vi "MWT.vi"() -> ()   [LabVIEW 2010]
uses:
  MWT_1.3.0_r1035/MultiWorm Tracker v1.3.0/data/MWT.dll
  <vilib>/vision/driver/NI_Vision_Acquisition_Software.lvlib
  <vilib>/vision/Image Controls.llb/IMAQ Image.ctl
  <vilib>/userDefined/High Color/IMAQdx.ctl
panel:
  in  "Turn on external triggering of camera":bool
  in  "User interface display slector":u16(ring)=2 items=["Raw Image", "Memory Image", "Fixed Image", "Nothing"]
  out "Auto-end in (s)":dbl
  out "error out 2":errorcluster
  in  "Minimum time between events(ms)":u32=2000
  in  "custom 1 timing array":dbl[](array[numeric])=[0.0]
  in  "puff timing array":dbl[](array[numeric])=[0.0]
  in  "tap timing array":dbl[](array[numeric])=[0.0]
  in  "custom 2 timing array":dbl[](array[numeric])=[0.0]
  in  "Tap Train Number":i32[][](array[numeric])=[[0, 1]]
  in  "Turn on Background division algorithm":bool
  in  "custom 2 fraction of time between is active":sgl[][](array[numeric])=[[0.0, 0.5]]
  in  "time between custom 2 onset":i32[][](array[numeric])=[[0, 50]]
  in  "custom 1 fraction of time between is active":sgl[][](array[numeric])=[[0.0, 0.5]]
  in  "time between custom 1 onset":i32[][](array[numeric])=[[0, 50]]
  in  "time between puff onset":i32[][](array[numeric])=[[0, 50]]
  in  "puff fraction of time between is active":sgl[][](array[numeric])=[[0.0, 0.5]]
  in  "time between tap onset":i32[][](array[numeric])=[[0, 10]]
  in  "tap fraction of time between is active":sgl[][](array[numeric])=[[0.0, 0.6]]
  in  "Turn on output aggregation?":bool=TRUE
  out "# Custom 2's Delivered":i32
  out "Time until Next Custom 2":dbl caption="No Custom 2s"
  in  "Custom 2 Signal-high lead up":i32=20
  in  "Custom 2 Signal-high duration":i32=50
  in  "Advanced Custom 2 Settings":bool
  in  "Custom 2 Stimulus Method":u16(ring) items=["Fixed Interval"=0, "Exponential Interval"=2, "Custom"=5]
  in  "Custom 2 Number":i32 caption="# of Puff events"
  in  "Custom 2 Interval":dbl caption="Custom Interval (s)"
  in  "Custom 2 Delay":dbl caption="Puff Onset Delay (s)" format="%#_4g"
  in  "Custom 2":bool
  out "Image Data Input Source":T1(ring)
  in  "Number of Image Adaptation Bands":i32=10
  out "error out":errorcluster
  in  "AVI path":path
  out "Auto-start in (s)":dbl
  in  "Auto-start delay (s)":i32
  in  "Raw Image Save Interval (s)":dbl
  in  "IMAQdx camera interface name":T2="cam0"
  out "Query for Interface?":bool=TRUE
  out "last acquired buffer":i32
  in  "Advanced Settings":bool
  out "# Custom 1's Delivered":i32
  out "Time until Next Custom 1":dbl caption="No Custom 1s"
  in  "Custom 1 Signal-high lead up":i32=20
  in  "Custom 1 Signal-high duration":i32=50
  out "Tracker Handle":i32=1
  out "IMAQ Session":refnum<k11>
  in  "Advanced Custom 1 Settings":bool
  in  "Custom 1 Stimulus Method":u16(ring) items=["Fixed Interval"=0, "Exponential Interval"=2, "Custom"=5]
  in  "Custom 1 Number":i32 caption="# of Puff events"
  in  "Custom 1 Interval":dbl caption="Custom Interval (s)"
  in  "Custom 1 Delay":dbl caption="Puff Onset Delay (s)" format="%#_4g"
  in  "Custom 1":bool
  in  "Image Binning":u16(ring)=1 items=["1"=1, "2"=2, "3"=3, "4"=4]
  in  "Contour?":bool
  in  "AFG resource name":refnum<k15>="COM1"
  out "Proccessing loop stopped?":bool
  in  "Object Border":i32=20
  out "AFG Settings":dbl[][](array[numeric])=[[0.0, 10.0, 1.0]]
  out "AFG instrument handle":refnum<k15> caption="instrument handle out"
  in  "Puff Signal-high lead up":i32=20
  in  "Puff Signal-high duration":i32=50
  in  "Frames of Adaptation":i32=10
  out "# Taps Delivered":i32
  out "# Puffs Delivered":i32
  in  "Skeletonize?":bool
  out "ROI Array":dbl[][](array[numeric])=[[0.0, 0.0, 2350.0, 1726.0, 0.0, 0.0]]
  out "Time until Next Puff":dbl caption="No Puffs"
  out "Seconds into Experiment":dbl
  out "Objects Found":i32
  in  "Bit Depth from Camera?":bool=TRUE
  in  "Image Bit Depth":u32=8
  in  "Advanced Puff Settings":bool
  in  "Graph Input 4":u16(ring)=9 items=["# objects", "# objects persisting", "Persistence", "Speed", "Angular Speed", "Length", "Relative Length", "Width", "Relative Width", "Aspect", "Relative Aspect", "Head Or Tail Angle", "Pixel Count"]
  in  "Graph Input 3":u16(ring)=3 items=["# objects", "# objects persisting", "Persistence", "Speed", "Angular Speed", "Length", "Relative Length", "Width", "Relative Width", "Aspect", "Relative Aspect", "Head Or Tail Angle", "Pixel Count"]
  in  "Graph Input 2":u16(ring)=1 items=["# objects", "# objects persisting", "Persistence", "Speed", "Angular Speed", "Length", "Relative Length", "Width", "Relative Width", "Aspect", "Relative Aspect", "Head Or Tail Angle", "Pixel Count"]
  in  "Graph Input":u16(ring) items=["# objects", "# objects persisting", "Persistence", "Speed", "Angular Speed", "Length", "Relative Length", "Width", "Relative Width", "Aspect", "Relative Aspect", "Head or Tail Angle", "Pixel Count"]
  out "XY Graph 4":cluster{sgl, sgl}[](graph)
  out "XY Graph 3":cluster{sgl, sgl}[](graph)
  out "XY Graph 2":cluster{sgl, sgl}[](graph)
  out "XY Graph":cluster{sgl, sgl}[](graph)
  out "Time until Next Tap":dbl caption="No Taps"
  in  "Puff Stimulus Method":u16(ring) items=["Fixed Interval"=0, "Exponential Interval"=2, "Custom"=5]
  in  "Tap Pulse Active downtime":i32=120
  in  "Tap Pulse Active duration":i32=120
  in  "Tap Signal-high duration":i32=100
  in  "Tap Signal-high lead up":i32=20
  out "seconds per frame":sgl
  out "error count":i32
  out "First-call":bool=TRUE
  in  "Run":bool
  in  "Adaptation Rate":i32=5 step=1
  out "Directory Exists?":bool
  in  "IMAQ Camera Interface Name":string="img0"
  in  "Display/Don't Display":bool=TRUE
  in  "What to display":u16(ring)=2 items=["Raw Image", "Memory Image", "Fixed Image"]
  out "Image":T3(plugin-control)
  in  "Stop":bool=TRUE
  in  "Set New Reference Object":bool
  in  "Clear Reference Object(s)":bool
  in  "Set Region of Interest":bool
  in  "Clear Region of Interest":bool
  in  "Load":bool
  in  "Save":bool
  in  "Advanced Tap Settings":bool
  in  "Tap Stimulus Method":u16(ring) items=["Fixed Interval"=0, "Exponential Interval"=2, "Custom"=5]
  in  "Puff Number":i32 caption="# of Puff events"
  in  "Puff Interval":dbl caption="Puff Interval (s)"
  in  "Puff Delay":dbl caption="Puff Onset Delay (s)"
  in  "Tap Number":i32 caption="# of Tap events" step=1
  in  "Tap Interval":dbl caption="Tap Interval (s)"
  in  "Tap Delay":dbl caption="Tap Onset Delay (s)"
  in  "Puff":bool
  in  "Tap":bool
  in  "Experiment Duration (s)":dbl
  in  "Prefix":string
  in  "Path":path
  in  "Object Size hysteresis (%)":dbl=10.0 min=0.5 max=99.5
  in  "Minimum Object Size (pixels)":i32=50
  in  "Maximum Object Size (pixels)":i32=6000
  in  "Fill Hysteresis (%)":dbl=50.0 min=0.5 max=99.5
  in  "Object Contrast (%)":dbl=10.0 min=0.5 max=99.5
  in  "Type of object to track":bool
  # "Display"
  # "Do not display"
  # "Region of Interest"
  # "Reference Object"
  # "Multi-Worm Tracker\nv1.3.0 r1035"
  # "Display"
  # "Object Tracker Settings"
  # "Contrast"
  # "Size"
  # "Bright Objects"
  # "Dark Objects"
  # "Data Ouput Settings"
  # "Stimulus Settings"
  # "On"
  # "On"
  # "On"
  # "On"
  # "Off"
  # "Off"
  # "Off"
  # "Off"
  # "Onset delay (s)"
  # "Interval (s)"
  # "Events (#)"
  # "Configuration"
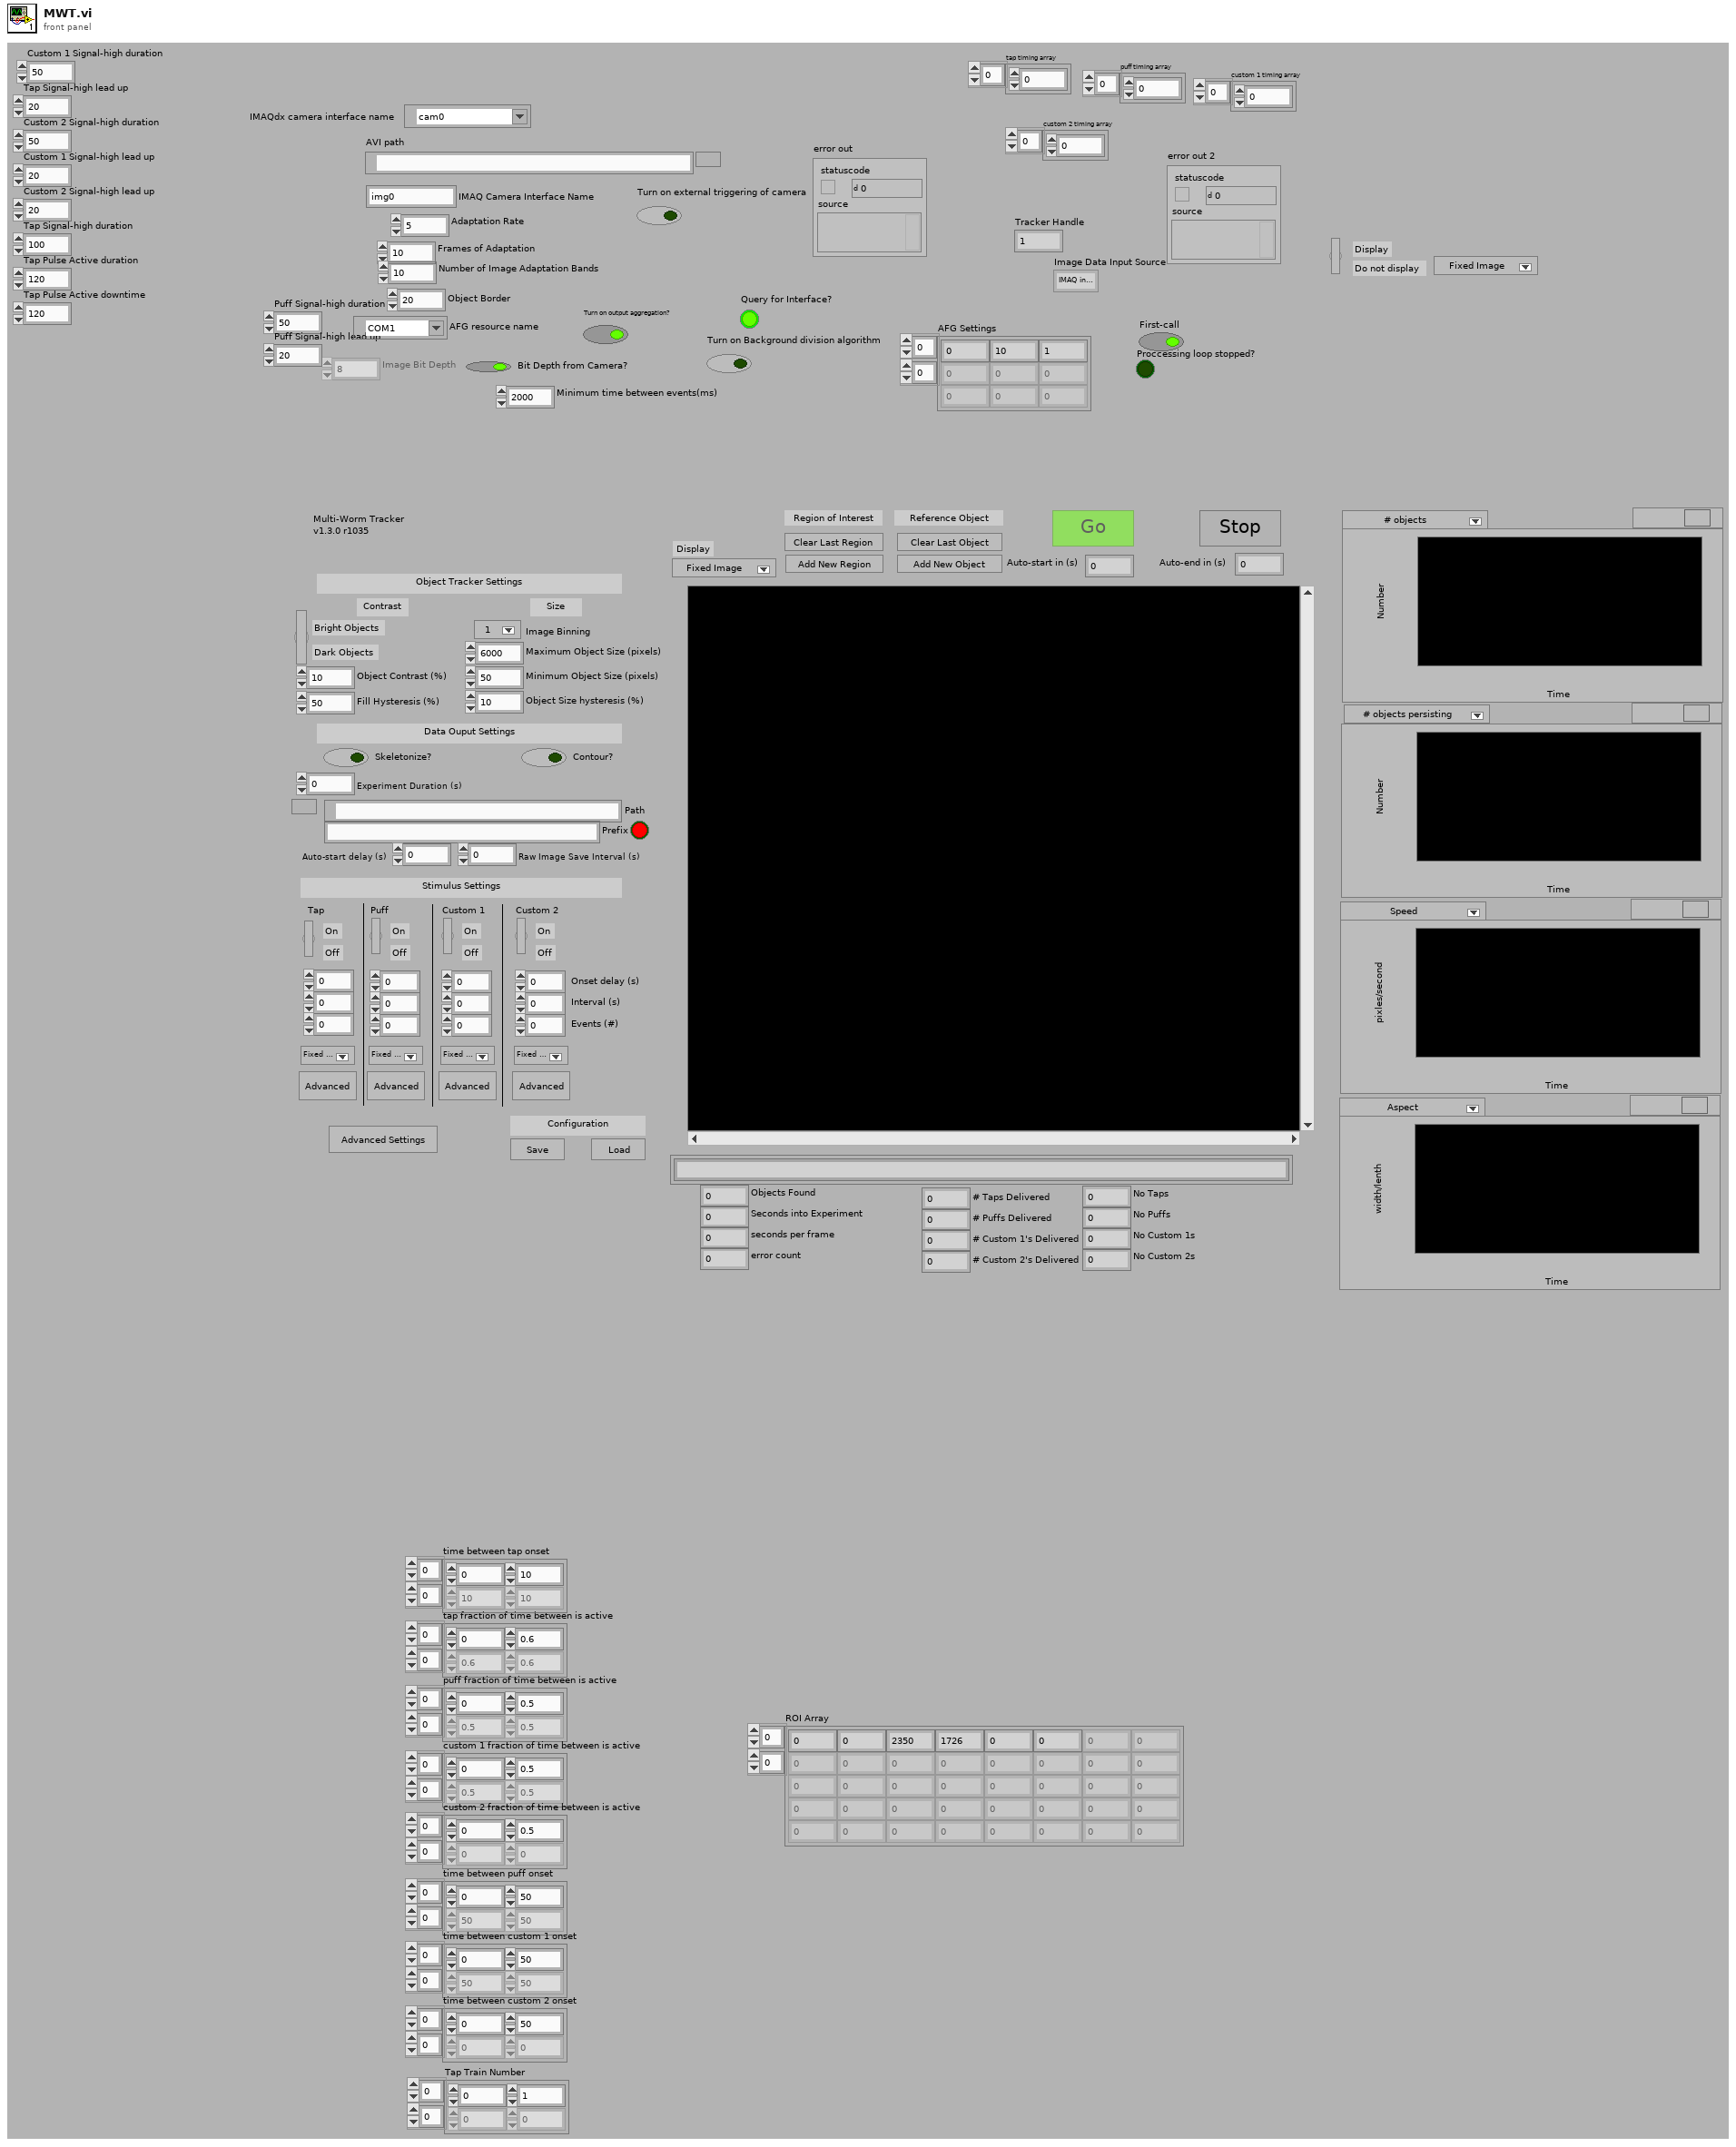
[diagram p1: front panel]
types:
  T1 = enum32{"IMAQ interface", "IMAQdx interface", "AVI file"}
  T2 = typedef "IMAQdx.ctl" = refnum<k21>
  T3 = typedef "IMAQ Image.ctl" = refnum<image>
  T4 = cluster{"Puff":refnum<vi>, "Puff Delay":refnum<vi>, "Puff Interval":refnum<vi>, "Puff Number":refnum<vi>, "Puff Stimulus Method":refnum<vi>}
  T5 = cluster{"Custom 2":refnum<vi>, "Custom 2 Delay":refnum<vi>, "Custom 2 Interval":refnum<vi>, "Custom 2 Number":refnum<vi>, "Custom 2 Stimulus Method":refnum<vi>}
  T6 = cluster{"Custom 1":refnum<vi>, "Custom 1 Delay":refnum<vi>, "Custom 1 Interval":refnum<vi>, "Custom 1 Number":refnum<vi>, "Custom 1 Stimulus Method":refnum<vi>}
  T7 = cluster{"Tap":refnum<vi>, "Tap Delay":refnum<vi>, "Tap Interval":refnum<vi>, "Tap Number":refnum<vi>, "Tap Stimulus Method":refnum<vi>}
  T8 = cluster{cluster{"Tap":refnum<vi>, "Tap Delay":refnum<vi>, "Tap Interval":refnum<vi>, "Tap Number":refnum<vi>, "Tap Stimulus Method":refnum<vi>}, cluster{"Puff":refnum<vi>, "Puff Delay":refnum<vi>, "Puff Interval":refnum<vi>, "Puff Number":refnum<vi>, "Puff Stimulus Method":refnum<vi>}, cluster{"Custom 1":refnum<vi>, "Custom 1 Delay":refnum<vi>, "Custom 1 Interval":refnum<vi>, "Custom 1 Number":refnum<vi>, "Custom 1 Stimulus Method":refnum<vi>}, cluster{"Custom 2":refnum<vi>, "Custom 2 Delay":refnum<vi>, "Custom 2 Interval":refnum<vi>, "Custom 2 Number":refnum<vi>, "Custom 2 Stimulus Method":refnum<vi>}}
  T9 = cluster{"Run":refnum<vi>, "Set Region of Interest":refnum<vi>, "Clear Region of Interest":refnum<vi>, "Clear Reference Object(s)":refnum<vi>, "Set New Reference Object":refnum<vi>, "Advanced Settings":refnum<vi>}
  T10 = cluster{"Path":refnum<vi>, "Prefix":refnum<vi>, "Type of object to track":refnum<vi>, "Object Contrast (%)":refnum<vi>, "Fill Hysteresis (%)":refnum<vi>, "Maximum Object Size (pixels)":refnum<vi>, "Minimum Object Size (pixels)":refnum<vi>, "Object Size hysteresis (%)":refnum<vi>, "Image Binning":refnum<vi>, "Contour?":refnum<vi>, "Skeletonize?":refnum<vi>, "Frames of Adaptation":refnum<vi>, "Adaptation Rate":refnum<vi>, "Object Border":refnum<vi>, "Image Bit Depth":refnum<vi>, "Bit Depth from Camera?":refnum<vi>, "AFG resource name":refnum<vi>, "IMAQ Camera Interface Name":refnum<vi>, "Auto-start delay (s)":refnum<vi>, "Number of Image Adaptation Bands":refnum<vi>, "Experiment Duration (s)":refnum<vi>, "Tap":refnum<vi>, "Tap Delay":refnum<vi>, "Tap Interval":refnum<vi>, "Tap Number":refnum<vi>, "Tap Stimulus Method":refnum<vi>, "Advanced Tap Settings":refnum<vi>, "Puff":refnum<vi>, "Puff Delay":refnum<vi>, "Puff Interval":refnum<vi>, "Puff Number":refnum<vi>, "Puff Stimulus Method":refnum<vi>, "Advanced Puff Settings":refnum<vi>, "Custom 1":refnum<vi>, "Custom 1 Delay":refnum<vi>, "Custom 1 Interval":refnum<vi>, "Custom 1 Number":refnum<vi>, "Custom 1 Stimulus Method":refnum<vi>, "Advanced Custom 1 Settings":refnum<vi>, "puff fraction of time between is active":refnum<vi>, "time between puff onset":refnum<vi>, "tap fraction of time between is active":refnum<vi>, "time between tap onset":refnum<vi>, "Tap Train Number":refnum<vi>, "custom 1 fraction of time between is active":refnum<vi>, "time between custom 1 onset":refnum<vi>, "Custom 2":refnum<vi>, "Custom 2 Delay":refnum<vi>, "Custom 2 Interval":refnum<vi>, "Custom 2 Number":refnum<vi>, "Custom 2 Stimulus Method":refnum<vi>, "Advanced Custom 2 Settings":refnum<vi>, "custom 2 fraction of time between is active":refnum<vi>, "time between custom 2 onset":refnum<vi>, "Save":refnum<vi>, "Load":refnum<vi>, "Raw Image Save Interval (s)":refnum<vi>, "Turn on output aggregation?":refnum<vi>, "Turn on Background division algorithm":refnum<vi>, "Turn on external triggering of camera":refnum<vi>}
  T11 = cluster{cluster{cluster{"Tap":refnum<vi>, "Tap Delay":refnum<vi>, "Tap Interval":refnum<vi>, "Tap Number":refnum<vi>, "Tap Stimulus Method":refnum<vi>}, cluster{"Puff":refnum<vi>, "Puff Delay":refnum<vi>, "Puff Interval":refnum<vi>, "Puff Number":refnum<vi>, "Puff Stimulus Method":refnum<vi>}, cluster{"Custom 1":refnum<vi>, "Custom 1 Delay":refnum<vi>, "Custom 1 Interval":refnum<vi>, "Custom 1 Number":refnum<vi>, "Custom 1 Stimulus Method":refnum<vi>}, cluster{"Custom 2":refnum<vi>, "Custom 2 Delay":refnum<vi>, "Custom 2 Interval":refnum<vi>, "Custom 2 Number":refnum<vi>, "Custom 2 Stimulus Method":refnum<vi>}}, cluster{"Path":refnum<vi>, "Prefix":refnum<vi>, "Type of object to track":refnum<vi>, "Object Contrast (%)":refnum<vi>, "Fill Hysteresis (%)":refnum<vi>, "Maximum Object Size (pixels)":refnum<vi>, "Minimum Object Size (pixels)":refnum<vi>, "Object Size hysteresis (%)":refnum<vi>, "Image Binning":refnum<vi>, "Contour?":refnum<vi>, "Skeletonize?":refnum<vi>, "Frames of Adaptation":refnum<vi>, "Adaptation Rate":refnum<vi>, "Object Border":refnum<vi>, "Image Bit Depth":refnum<vi>, "Bit Depth from Camera?":refnum<vi>, "AFG resource name":refnum<vi>, "IMAQ Camera Interface Name":refnum<vi>, "Auto-start delay (s)":refnum<vi>, "Number of Image Adaptation Bands":refnum<vi>, "Experiment Duration (s)":refnum<vi>, "Tap":refnum<vi>, "Tap Delay":refnum<vi>, "Tap Interval":refnum<vi>, "Tap Number":refnum<vi>, "Tap Stimulus Method":refnum<vi>, "Advanced Tap Settings":refnum<vi>, "Puff":refnum<vi>, "Puff Delay":refnum<vi>, "Puff Interval":refnum<vi>, "Puff Number":refnum<vi>, "Puff Stimulus Method":refnum<vi>, "Advanced Puff Settings":refnum<vi>, "Custom 1":refnum<vi>, "Custom 1 Delay":refnum<vi>, "Custom 1 Interval":refnum<vi>, "Custom 1 Number":refnum<vi>, "Custom 1 Stimulus Method":refnum<vi>, "Advanced Custom 1 Settings":refnum<vi>, "puff fraction of time between is active":refnum<vi>, "time between puff onset":refnum<vi>, "tap fraction of time between is active":refnum<vi>, "time between tap onset":refnum<vi>, "Tap Train Number":refnum<vi>, "custom 1 fraction of time between is active":refnum<vi>, "time between custom 1 onset":refnum<vi>, "Custom 2":refnum<vi>, "Custom 2 Delay":refnum<vi>, "Custom 2 Interval":refnum<vi>, "Custom 2 Number":refnum<vi>, "Custom 2 Stimulus Method":refnum<vi>, "Advanced Custom 2 Settings":refnum<vi>, "custom 2 fraction of time between is active":refnum<vi>, "time between custom 2 onset":refnum<vi>, "Save":refnum<vi>, "Load":refnum<vi>, "Raw Image Save Interval (s)":refnum<vi>, "Turn on output aggregation?":refnum<vi>, "Turn on Background division algorithm":refnum<vi>, "Turn on external triggering of camera":refnum<vi>}, cluster{"Run":refnum<vi>, "Set Region of Interest":refnum<vi>, "Clear Region of Interest":refnum<vi>, "Clear Reference Object(s)":refnum<vi>, "Set New Reference Object":refnum<vi>, "Advanced Settings":refnum<vi>}}
  T12 = cluster{"Value":bool, "Value":dbl, "Value":dbl, "Value":i32, "Value":u16}
  T13 = typedef "AviRefnum.ctl" = refnum<k1>
  T14 = cluster{"IMAQ Session Out":refnum<k11>, "Avi Refnum":T13, "Value":enum32{"IMAQ interface", "IMAQdx interface", "AVI file"}, "Session Out":T2, "Value":bool}
  T15 = cluster{"IMAQ Session":refnum<k11>, "AVI Refnum":refnum<k1>, "Image Data Input Source":enum32{"IMAQ interface", "IMAQdx interface", "AVI file", "MMF File"}, cluster{"IMAQ Name":string, "IMAQDx Session":T2, "AVI/MMF Path":path}, "error?":bool, "use extrenal trigger":bool, "SR handle":u32}
  T16 = enum32{"IMAQ interface", "IMAQdx interface", "AVI file", "MMF File"}
  T17 = cluster{"IMAQ Name":string, "IMAQDx Session":T2, "AVI/MMF Path":path}
  T18 = cluster{"IMAQ Session":refnum<k11>, "AVI Refnum":refnum<k1>, "Image Data Input Source":enum32{"IMAQ interface", "IMAQdx interface", "AVI file", "MMF File"}, "SR handle":u32}
  T19 = cluster{"IMAQ Session":refnum<k11>, "AVI Refnum":refnum<k1>, "Image Data Input Source":enum32{"IMAQ interface", "IMAQdx interface", "AVI file", "MMF File"}, "IMAQDx Session":T2, "Value":bool, "SR handle":u32}
  T20 = typedef "Image Type" = u32
  T21 = cluster{"Value":path, "Value":string, "Value":bool, "Value":dbl, "Value":dbl, "Value":i32, "Value":i32, "Value":dbl, "Value":u16, "Value":bool, "Value":bool, "Value":i32, "Value":i32, "Value":i32, "Value":u32, "Value":i32, "Value":bool}
  T22 = cluster{"AFG Settings":dbl[][], "tap timing array":dbl[], "puff timing array":dbl[], "custom timing array":dbl[], "custom 2 timing array":dbl[], cluster{cluster{"Tap":refnum<vi>, "Tap Delay":refnum<vi>, "Tap Interval":refnum<vi>, "Tap Number":refnum<vi>, "Tap Stimulus Method":refnum<vi>}, cluster{"Puff":refnum<vi>, "Puff Delay":refnum<vi>, "Puff Interval":refnum<vi>, "Puff Number":refnum<vi>, "Puff Stimulus Method":refnum<vi>}, cluster{"Custom 1":refnum<vi>, "Custom 1 Delay":refnum<vi>, "Custom 1 Interval":refnum<vi>, "Custom 1 Number":refnum<vi>, "Custom 1 Stimulus Method":refnum<vi>}, cluster{"Custom 2":refnum<vi>, "Custom 2 Delay":refnum<vi>, "Custom 2 Interval":refnum<vi>, "Custom 2 Number":refnum<vi>, "Custom 2 Stimulus Method":refnum<vi>}}, cluster{"Path":refnum<vi>, "Prefix":refnum<vi>, "Type of object to track":refnum<vi>, "Object Contrast (%)":refnum<vi>, "Fill Hysteresis (%)":refnum<vi>, "Maximum Object Size (pixels)":refnum<vi>, "Minimum Object Size (pixels)":refnum<vi>, "Object Size hysteresis (%)":refnum<vi>, "Image Binning":refnum<vi>, "Contour?":refnum<vi>, "Skeletonize?":refnum<vi>, "Frames of Adaptation":refnum<vi>, "Adaptation Rate":refnum<vi>, "Object Border":refnum<vi>, "Image Bit Depth":refnum<vi>, "Bit Depth from Camera?":refnum<vi>, "AFG resource name":refnum<vi>, "IMAQ Camera Interface Name":refnum<vi>, "Auto-start delay (s)":refnum<vi>, "Number of Image Adaptation Bands":refnum<vi>, "Experiment Duration (s)":refnum<vi>, "Tap":refnum<vi>, "Tap Delay":refnum<vi>, "Tap Interval":refnum<vi>, "Tap Number":refnum<vi>, "Tap Stimulus Method":refnum<vi>, "Advanced Tap Settings":refnum<vi>, "Puff":refnum<vi>, "Puff Delay":refnum<vi>, "Puff Interval":refnum<vi>, "Puff Number":refnum<vi>, "Puff Stimulus Method":refnum<vi>, "Advanced Puff Settings":refnum<vi>, "Custom 1":refnum<vi>, "Custom 1 Delay":refnum<vi>, "Custom 1 Interval":refnum<vi>, "Custom 1 Number":refnum<vi>, "Custom 1 Stimulus Method":refnum<vi>, "Advanced Custom 1 Settings":refnum<vi>, "puff fraction of time between is active":refnum<vi>, "time between puff onset":refnum<vi>, "tap fraction of time between is active":refnum<vi>, "time between tap onset":refnum<vi>, "Tap Train Number":refnum<vi>, "custom 1 fraction of time between is active":refnum<vi>, "time between custom 1 onset":refnum<vi>, "Custom 2":refnum<vi>, "Custom 2 Delay":refnum<vi>, "Custom 2 Interval":refnum<vi>, "Custom 2 Number":refnum<vi>, "Custom 2 Stimulus Method":refnum<vi>, "Advanced Custom 2 Settings":refnum<vi>, "custom 2 fraction of time between is active":refnum<vi>, "time between custom 2 onset":refnum<vi>, "Save":refnum<vi>, "Load":refnum<vi>, "Raw Image Save Interval (s)":refnum<vi>, "Turn on output aggregation?":refnum<vi>, "Turn on Background division algorithm":refnum<vi>, "Turn on external triggering of camera":refnum<vi>}, "output values cluster":cluster{"Value":bool, "Value":dbl, "Value":dbl, "Value":dbl, "Value":u16}, "output values cluster":cluster{"Value":bool, "Value":dbl, "Value":dbl, "Value":dbl, "Value":u16}, "output values cluster":cluster{"Value":bool, "Value":dbl, "Value":dbl, "Value":dbl, "Value":u16}, "output values cluster":cluster{"Value":bool, "Value":dbl, "Value":dbl, "Value":dbl, "Value":u16}}
  T23 = cluster{cluster{"IMAQ Session":refnum<k11>, "AVI Refnum":refnum<k1>, "Image Data Input Source":enum32{"IMAQ interface", "IMAQdx interface", "AVI file", "MMF File"}, "IMAQDx Session":T2, "Value":bool, "SR handle":u32}, "Value":i32, "Value":i32}
  T24 = cluster{"output values cluster":cluster{"Value":bool, "Value":dbl, "Value":dbl, "Value":dbl, "Value":u16}, "Output Array":dbl[], "output values cluster":cluster{"Value":bool, "Value":dbl, "Value":dbl, "Value":dbl, "Value":u16}, "Output Array":dbl[], "output values cluster":cluster{"Value":bool, "Value":dbl, "Value":dbl, "Value":dbl, "Value":u16}, "Output Array":dbl[], "AFG Settings":dbl[][], "output values cluster":cluster{"Value":bool, "Value":dbl, "Value":dbl, "Value":dbl, "Value":u16}, "Output Array":dbl[]}
  T25 = cluster{cluster{cluster{"IMAQ Session":refnum<k11>, "AVI Refnum":refnum<k1>, "Image Data Input Source":enum32{"IMAQ interface", "IMAQdx interface", "AVI file", "MMF File"}, "IMAQDx Session":T2, "Value":bool, "SR handle":u32}, "Value":i32, "Value":i32}, cluster{"Run":refnum<vi>, "Set Region of Interest":refnum<vi>, "Clear Region of Interest":refnum<vi>, "Clear Reference Object(s)":refnum<vi>, "Set New Reference Object":refnum<vi>, "Advanced Settings":refnum<vi>}, "Image Bit Depth":u32}
  T26 = cluster{"Value":bool, "Value":dbl, "Value":dbl, "Value":dbl, "Value":u16}
  T27 = cluster{cluster{cluster{"IMAQ Session":refnum<k11>, "AVI Refnum":refnum<k1>, "Image Data Input Source":enum32{"IMAQ interface", "IMAQdx interface", "AVI file", "MMF File"}, "IMAQDx Session":T2, "Value":bool, "SR handle":u32}, "Value":i32, "Value":i32}, cluster{"Path":refnum<vi>, "Prefix":refnum<vi>, "Type of object to track":refnum<vi>, "Object Contrast (%)":refnum<vi>, "Fill Hysteresis (%)":refnum<vi>, "Maximum Object Size (pixels)":refnum<vi>, "Minimum Object Size (pixels)":refnum<vi>, "Object Size hysteresis (%)":refnum<vi>, "Image Binning":refnum<vi>, "Contour?":refnum<vi>, "Skeletonize?":refnum<vi>, "Frames of Adaptation":refnum<vi>, "Adaptation Rate":refnum<vi>, "Object Border":refnum<vi>, "Image Bit Depth":refnum<vi>, "Bit Depth from Camera?":refnum<vi>, "AFG resource name":refnum<vi>, "IMAQ Camera Interface Name":refnum<vi>, "Auto-start delay (s)":refnum<vi>, "Number of Image Adaptation Bands":refnum<vi>, "Experiment Duration (s)":refnum<vi>, "Tap":refnum<vi>, "Tap Delay":refnum<vi>, "Tap Interval":refnum<vi>, "Tap Number":refnum<vi>, "Tap Stimulus Method":refnum<vi>, "Advanced Tap Settings":refnum<vi>, "Puff":refnum<vi>, "Puff Delay":refnum<vi>, "Puff Interval":refnum<vi>, "Puff Number":refnum<vi>, "Puff Stimulus Method":refnum<vi>, "Advanced Puff Settings":refnum<vi>, "Custom 1":refnum<vi>, "Custom 1 Delay":refnum<vi>, "Custom 1 Interval":refnum<vi>, "Custom 1 Number":refnum<vi>, "Custom 1 Stimulus Method":refnum<vi>, "Advanced Custom 1 Settings":refnum<vi>, "puff fraction of time between is active":refnum<vi>, "time between puff onset":refnum<vi>, "tap fraction of time between is active":refnum<vi>, "time between tap onset":refnum<vi>, "Tap Train Number":refnum<vi>, "custom 1 fraction of time between is active":refnum<vi>, "time between custom 1 onset":refnum<vi>, "Custom 2":refnum<vi>, "Custom 2 Delay":refnum<vi>, "Custom 2 Interval":refnum<vi>, "Custom 2 Number":refnum<vi>, "Custom 2 Stimulus Method":refnum<vi>, "Advanced Custom 2 Settings":refnum<vi>, "custom 2 fraction of time between is active":refnum<vi>, "time between custom 2 onset":refnum<vi>, "Save":refnum<vi>, "Load":refnum<vi>, "Raw Image Save Interval (s)":refnum<vi>, "Turn on output aggregation?":refnum<vi>, "Turn on Background division algorithm":refnum<vi>, "Turn on external triggering of camera":refnum<vi>}, "ROI Array":dbl[][], "settings value cluster":cluster{"Value":path, "Value":string, "Value":bool, "Value":dbl, "Value":dbl, "Value":i32, "Value":i32, "Value":dbl, "Value":u16, "Value":bool, "Value":bool, "Value":i32, "Value":i32, "Value":i32, "Value":u32, "Value":i32, "Value":bool}, "AFG Settings":dbl[][], "Output Array":dbl[], "Output Array":dbl[], "Output Array":dbl[], "Output Array":dbl[]}
  T28 = cluster{"Output  ROI Array":dbl[][], "settings value cluster":cluster{"Value":path, "Value":string, "Value":bool, "Value":dbl, "Value":dbl, "Value":i32, "Value":i32, "Value":dbl, "Value":u16, "Value":bool, "Value":bool, "Value":i32, "Value":i32, "Value":i32, "Value":u32, "Value":i32, "Value":bool}, "AFG Settings":dbl[][], "tap timing array":dbl[], "puff timing array":dbl[], "custom timing array":dbl[], "custom 2 timing array":dbl[]}
  T29 = cluster{cluster{"Path":refnum<vi>, "Prefix":refnum<vi>, "Type of object to track":refnum<vi>, "Object Contrast (%)":refnum<vi>, "Fill Hysteresis (%)":refnum<vi>, "Maximum Object Size (pixels)":refnum<vi>, "Minimum Object Size (pixels)":refnum<vi>, "Object Size hysteresis (%)":refnum<vi>, "Image Binning":refnum<vi>, "Contour?":refnum<vi>, "Skeletonize?":refnum<vi>, "Frames of Adaptation":refnum<vi>, "Adaptation Rate":refnum<vi>, "Object Border":refnum<vi>, "Image Bit Depth":refnum<vi>, "Bit Depth from Camera?":refnum<vi>, "AFG resource name":refnum<vi>, "IMAQ Camera Interface Name":refnum<vi>, "Auto-start delay (s)":refnum<vi>, "Number of Image Adaptation Bands":refnum<vi>, "Experiment Duration (s)":refnum<vi>, "Tap":refnum<vi>, "Tap Delay":refnum<vi>, "Tap Interval":refnum<vi>, "Tap Number":refnum<vi>, "Tap Stimulus Method":refnum<vi>, "Advanced Tap Settings":refnum<vi>, "Puff":refnum<vi>, "Puff Delay":refnum<vi>, "Puff Interval":refnum<vi>, "Puff Number":refnum<vi>, "Puff Stimulus Method":refnum<vi>, "Advanced Puff Settings":refnum<vi>, "Custom 1":refnum<vi>, "Custom 1 Delay":refnum<vi>, "Custom 1 Interval":refnum<vi>, "Custom 1 Number":refnum<vi>, "Custom 1 Stimulus Method":refnum<vi>, "Advanced Custom 1 Settings":refnum<vi>, "puff fraction of time between is active":refnum<vi>, "time between puff onset":refnum<vi>, "tap fraction of time between is active":refnum<vi>, "time between tap onset":refnum<vi>, "Tap Train Number":refnum<vi>, "custom 1 fraction of time between is active":refnum<vi>, "time between custom 1 onset":refnum<vi>, "Custom 2":refnum<vi>, "Custom 2 Delay":refnum<vi>, "Custom 2 Interval":refnum<vi>, "Custom 2 Number":refnum<vi>, "Custom 2 Stimulus Method":refnum<vi>, "Advanced Custom 2 Settings":refnum<vi>, "custom 2 fraction of time between is active":refnum<vi>, "time between custom 2 onset":refnum<vi>, "Save":refnum<vi>, "Load":refnum<vi>, "Raw Image Save Interval (s)":refnum<vi>, "Turn on output aggregation?":refnum<vi>, "Turn on Background division algorithm":refnum<vi>, "Turn on external triggering of camera":refnum<vi>}, cluster{"IMAQ Session":refnum<k11>, "AVI Refnum":refnum<k1>, "Image Data Input Source":enum32{"IMAQ interface", "IMAQdx interface", "AVI file", "MMF File"}, "IMAQDx Session":T2, "Value":bool, "SR handle":u32}}
  T30 = cluster{cluster{cluster{"IMAQ Session":refnum<k11>, "AVI Refnum":refnum<k1>, "Image Data Input Source":enum32{"IMAQ interface", "IMAQdx interface", "AVI file", "MMF File"}, "IMAQDx Session":T2, "Value":bool, "SR handle":u32}, "Value":i32, "Value":i32}, "Image Binning":u16, "Value":u16}
  T31 = cluster{"Acquired Buffer Number":i32, "return type":i32, "destination":i16[][]}
  T32 = cluster{cluster{cluster{"IMAQ Session":refnum<k11>, "AVI Refnum":refnum<k1>, "Image Data Input Source":enum32{"IMAQ interface", "IMAQdx interface", "AVI file", "MMF File"}, "IMAQDx Session":T2, "Value":bool, "SR handle":u32}, "Value":i32, "Value":i32}, "ROI Array":dbl[][], "Value":bool, cluster{"Path":refnum<vi>, "Prefix":refnum<vi>, "Type of object to track":refnum<vi>, "Object Contrast (%)":refnum<vi>, "Fill Hysteresis (%)":refnum<vi>, "Maximum Object Size (pixels)":refnum<vi>, "Minimum Object Size (pixels)":refnum<vi>, "Object Size hysteresis (%)":refnum<vi>, "Image Binning":refnum<vi>, "Contour?":refnum<vi>, "Skeletonize?":refnum<vi>, "Frames of Adaptation":refnum<vi>, "Adaptation Rate":refnum<vi>, "Object Border":refnum<vi>, "Image Bit Depth":refnum<vi>, "Bit Depth from Camera?":refnum<vi>, "AFG resource name":refnum<vi>, "IMAQ Camera Interface Name":refnum<vi>, "Auto-start delay (s)":refnum<vi>, "Number of Image Adaptation Bands":refnum<vi>, "Experiment Duration (s)":refnum<vi>, "Tap":refnum<vi>, "Tap Delay":refnum<vi>, "Tap Interval":refnum<vi>, "Tap Number":refnum<vi>, "Tap Stimulus Method":refnum<vi>, "Advanced Tap Settings":refnum<vi>, "Puff":refnum<vi>, "Puff Delay":refnum<vi>, "Puff Interval":refnum<vi>, "Puff Number":refnum<vi>, "Puff Stimulus Method":refnum<vi>, "Advanced Puff Settings":refnum<vi>, "Custom 1":refnum<vi>, "Custom 1 Delay":refnum<vi>, "Custom 1 Interval":refnum<vi>, "Custom 1 Number":refnum<vi>, "Custom 1 Stimulus Method":refnum<vi>, "Advanced Custom 1 Settings":refnum<vi>, "puff fraction of time between is active":refnum<vi>, "time between puff onset":refnum<vi>, "tap fraction of time between is active":refnum<vi>, "time between tap onset":refnum<vi>, "Tap Train Number":refnum<vi>, "custom 1 fraction of time between is active":refnum<vi>, "time between custom 1 onset":refnum<vi>, "Custom 2":refnum<vi>, "Custom 2 Delay":refnum<vi>, "Custom 2 Interval":refnum<vi>, "Custom 2 Number":refnum<vi>, "Custom 2 Stimulus Method":refnum<vi>, "Advanced Custom 2 Settings":refnum<vi>, "custom 2 fraction of time between is active":refnum<vi>, "time between custom 2 onset":refnum<vi>, "Save":refnum<vi>, "Load":refnum<vi>, "Raw Image Save Interval (s)":refnum<vi>, "Turn on output aggregation?":refnum<vi>, "Turn on Background division algorithm":refnum<vi>, "Turn on external triggering of camera":refnum<vi>}, cluster{"Run":refnum<vi>, "Set Region of Interest":refnum<vi>, "Clear Region of Interest":refnum<vi>, "Clear Reference Object(s)":refnum<vi>, "Set New Reference Object":refnum<vi>, "Advanced Settings":refnum<vi>}, "Directory Exists?":refnum<vi>}
  T33 = cluster{cluster{"IMAQ Session":refnum<k11>, "AVI Refnum":refnum<k1>, "Image Data Input Source":enum32{"IMAQ interface", "IMAQdx interface", "AVI file", "MMF File"}, "IMAQDx Session":T2, "Value":bool, "SR handle":u32}, i32}
  T34 = cluster{"tap timing array":dbl[], "puff timing array":dbl[], "custom timing array":dbl[], "custom 2 timing array":dbl[]}
  T35 = cluster{"width":u32, "height":u32, "framesPerSecond":u32, "compressionFilter":string, "hasData":bool}
  T36 = cluster{cluster{"IMAQ Session":refnum<k11>, "AVI Refnum":refnum<k1>, "Image Data Input Source":enum32{"IMAQ interface", "IMAQdx interface", "AVI file", "MMF File"}, "IMAQDx Session":T2, "Value":bool, "SR handle":u32}, "Value":i32}
  T37 = cluster{cluster{cluster{"IMAQ Session":refnum<k11>, "AVI Refnum":refnum<k1>, "Image Data Input Source":enum32{"IMAQ interface", "IMAQdx interface", "AVI file", "MMF File"}, "IMAQDx Session":T2, "Value":bool, "SR handle":u32}, "Value":i32}, "Value":i32, "Value":i32, "Value":u16, "Image":T3}
  T38 = cluster{cluster{"IMAQ Session":refnum<k11>, "AVI Refnum":refnum<k1>, "Image Data Input Source":enum32{"IMAQ interface", "IMAQdx interface", "AVI file", "MMF File"}, "IMAQDx Session":T2, "Value":bool, "SR handle":u32}, "Acquired Buffer Number":u32}
  T39 = cluster{cluster{"Path":refnum<vi>, "Prefix":refnum<vi>, "Type of object to track":refnum<vi>, "Object Contrast (%)":refnum<vi>, "Fill Hysteresis (%)":refnum<vi>, "Maximum Object Size (pixels)":refnum<vi>, "Minimum Object Size (pixels)":refnum<vi>, "Object Size hysteresis (%)":refnum<vi>, "Image Binning":refnum<vi>, "Contour?":refnum<vi>, "Skeletonize?":refnum<vi>, "Frames of Adaptation":refnum<vi>, "Adaptation Rate":refnum<vi>, "Object Border":refnum<vi>, "Image Bit Depth":refnum<vi>, "Bit Depth from Camera?":refnum<vi>, "AFG resource name":refnum<vi>, "IMAQ Camera Interface Name":refnum<vi>, "Auto-start delay (s)":refnum<vi>, "Number of Image Adaptation Bands":refnum<vi>, "Experiment Duration (s)":refnum<vi>, "Tap":refnum<vi>, "Tap Delay":refnum<vi>, "Tap Interval":refnum<vi>, "Tap Number":refnum<vi>, "Tap Stimulus Method":refnum<vi>, "Advanced Tap Settings":refnum<vi>, "Puff":refnum<vi>, "Puff Delay":refnum<vi>, "Puff Interval":refnum<vi>, "Puff Number":refnum<vi>, "Puff Stimulus Method":refnum<vi>, "Advanced Puff Settings":refnum<vi>, "Custom 1":refnum<vi>, "Custom 1 Delay":refnum<vi>, "Custom 1 Interval":refnum<vi>, "Custom 1 Number":refnum<vi>, "Custom 1 Stimulus Method":refnum<vi>, "Advanced Custom 1 Settings":refnum<vi>, "puff fraction of time between is active":refnum<vi>, "time between puff onset":refnum<vi>, "tap fraction of time between is active":refnum<vi>, "time between tap onset":refnum<vi>, "Tap Train Number":refnum<vi>, "custom 1 fraction of time between is active":refnum<vi>, "time between custom 1 onset":refnum<vi>, "Custom 2":refnum<vi>, "Custom 2 Delay":refnum<vi>, "Custom 2 Interval":refnum<vi>, "Custom 2 Number":refnum<vi>, "Custom 2 Stimulus Method":refnum<vi>, "Advanced Custom 2 Settings":refnum<vi>, "custom 2 fraction of time between is active":refnum<vi>, "time between custom 2 onset":refnum<vi>, "Save":refnum<vi>, "Load":refnum<vi>, "Raw Image Save Interval (s)":refnum<vi>, "Turn on output aggregation?":refnum<vi>, "Turn on Background division algorithm":refnum<vi>, "Turn on external triggering of camera":refnum<vi>}, "appended path":path, "ROI Array":dbl[][], "AFG Settings":dbl[][], "tap timing array":dbl[], "puff timing array":dbl[], "custom timing array":dbl[], "custom 2 timing array":dbl[]}
  T40 = cluster{cluster{"IMAQ Session":refnum<k11>, "AVI Refnum":refnum<k1>, "Image Data Input Source":enum32{"IMAQ interface", "IMAQdx interface", "AVI file", "MMF File"}, "IMAQDx Session":T2, "Value":bool, "SR handle":u32}, "Acquired Buffer Number":i32}
  T41 = cluster{"Graph Input":refnum<vi>, "Graph Input 2":refnum<vi>, "Graph Input 3":refnum<vi>, "Graph Input 4":refnum<vi>, "XY Graph":refnum<vi>, "XY Graph 2":refnum<vi>, "XY Graph 3":refnum<vi>, "XY Graph 4":refnum<vi>}
  T42 = cluster{"Value":sgl[][], "Value":i32[][], "Value":i32[][]}
  T43 = cluster{cluster{sgl, sgl}[], cluster{sgl, sgl}[], cluster{sgl, sgl}[], cluster{sgl, sgl}[], cluster{sgl, sgl}[], cluster{sgl, sgl}[], cluster{sgl, sgl}[], cluster{sgl, sgl}[], cluster{sgl, sgl}[], cluster{sgl, sgl}[], cluster{sgl, sgl}[], cluster{sgl, sgl}[], cluster{sgl, sgl}[]}
  T44 = cluster{"custom timing array":dbl[], i32, i32, "Value":bool, i32, "stimulus settings":cluster{"outy3":sgl, "outy3":i32}}
  T45 = cluster{"custom 2 timing array":dbl[], i32, i32, "Value":bool, i32, "stimulus settings":cluster{"outy3":sgl, "outy3":i32}}
  T46 = cluster{"puff timing array":dbl[], i32, i32, "Value":bool, i32, "stimulus settings":cluster{"outy3":sgl, "outy3":i32}}
  T47 = cluster{"tap timing array":dbl[], i32, i32, "Value":bool, i32, "stimulus settings":cluster{"outy3":sgl, "outy3":i32, "Value":i32}}
  T48 = cluster{u32, "millisecond timer value":u32, "millisecond timer value":u32, "Value":u32}
  T49 = cluster{cluster{u32, "millisecond timer value":u32, "millisecond timer value":u32, "Value":u32}, "Time until Next Tap":refnum<vi>, cluster{"tap timing array":dbl[], i32, i32, "Value":bool, i32, "stimulus settings":cluster{"outy3":sgl, "outy3":i32, "Value":i32}}}
  T50 = cluster{cluster{u32, "millisecond timer value":u32, "millisecond timer value":u32, "Value":u32}, "Time until Next Puff":refnum<vi>, cluster{"puff timing array":dbl[], i32, i32, "Value":bool, i32, "stimulus settings":cluster{"outy3":sgl, "outy3":i32}}}
  T51 = cluster{cluster{u32, "millisecond timer value":u32, "millisecond timer value":u32, "Value":u32}, "Time until Next Custom 1":refnum<vi>, cluster{"custom timing array":dbl[], i32, i32, "Value":bool, i32, "stimulus settings":cluster{"outy3":sgl, "outy3":i32}}}
  T52 = cluster{cluster{u32, "millisecond timer value":u32, "millisecond timer value":u32, "Value":u32}, "Time until Next Custom 2":refnum<vi>, cluster{"custom 2 timing array":dbl[], i32, i32, "Value":bool, i32, "stimulus settings":cluster{"outy3":sgl, "outy3":i32}}}
  T53 = cluster{"millisecond timer value":u32, "millisecond timer value":u32, i32, sgl, "Data Cluster":cluster{cluster{sgl, sgl}[], cluster{sgl, sgl}[], cluster{sgl, sgl}[], cluster{sgl, sgl}[], cluster{sgl, sgl}[], cluster{sgl, sgl}[], cluster{sgl, sgl}[], cluster{sgl, sgl}[], cluster{sgl, sgl}[], cluster{sgl, sgl}[], cluster{sgl, sgl}[], cluster{sgl, sgl}[], cluster{sgl, sgl}[]}, "Value":i32, cluster{"Graph Input":refnum<vi>, "Graph Input 2":refnum<vi>, "Graph Input 3":refnum<vi>, "Graph Input 4":refnum<vi>, "XY Graph":refnum<vi>, "XY Graph 2":refnum<vi>, "XY Graph 3":refnum<vi>, "XY Graph 4":refnum<vi>}}
  T54 = cluster{i32, "Tap Number":i32, "Elapsed Time":i32}
  T55 = cluster{"Elapsed Time":i32, "Data Cluster":cluster{cluster{sgl, sgl}[], cluster{sgl, sgl}[], cluster{sgl, sgl}[], cluster{sgl, sgl}[], cluster{sgl, sgl}[], cluster{sgl, sgl}[], cluster{sgl, sgl}[], cluster{sgl, sgl}[], cluster{sgl, sgl}[], cluster{sgl, sgl}[], cluster{sgl, sgl}[], cluster{sgl, sgl}[], cluster{sgl, sgl}[]}}
  T56 = cluster{i32, "Value":i32, "Value":u16, sgl, "Value":u16, "Value":bool, "Value":u32, "Image Out":T3, "Image Pixels (I16)":i16[][], i32[]}
  T57 = cluster{"return value":i32, "return value":i32, "Image Pixels (I16) out":i16[][], "coordinates":i32[]}
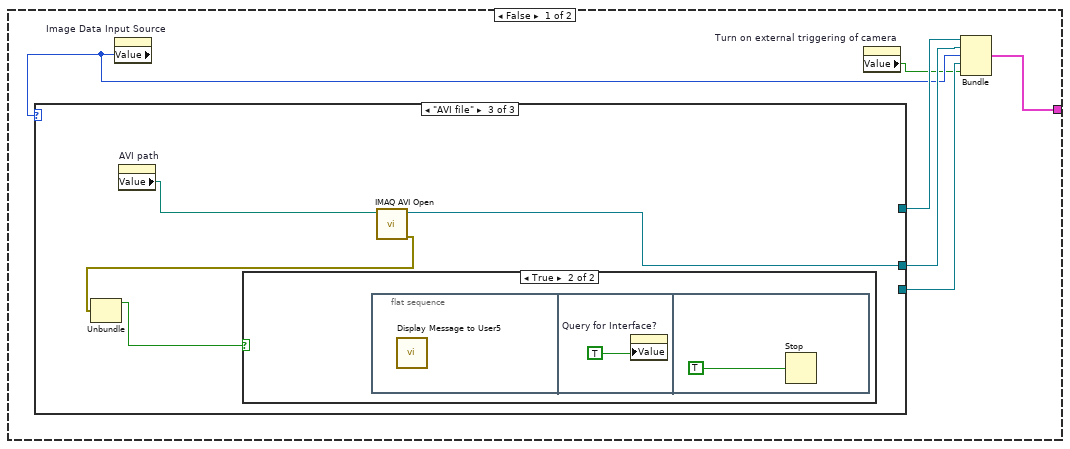
[diagram p2: hidden frame]
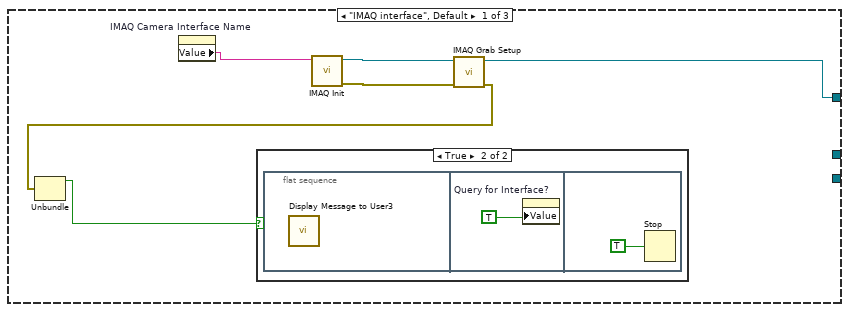
[diagram p3: hidden frame]
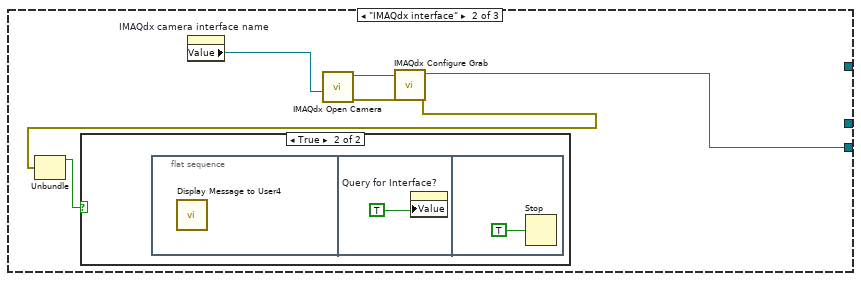
[diagram p5: hidden frame]
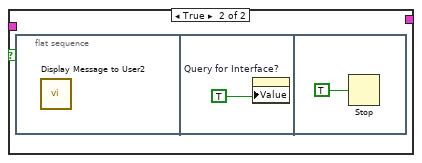
[diagram p8: hidden frame]
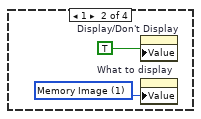
[diagram p11: hidden frame]
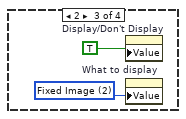
[diagram p12: hidden frame]
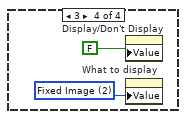
[diagram p13: hidden frame]
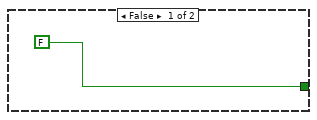
[diagram p14: hidden frame]
diagram:
  w3 = cluster{sgl, sgl}[] [] ("XY Graph")
  w24 = 0
  # "Stimulus counter trigger arrays"
  # "Stimulus event timing arrays"
  # "Copyright (C) 2007 - 2010 Howard Hughes Medical Institute\nCopyright (C) 2007 - 2010 Rex A. Kerr, Nicholas A. Swierczek\n \nThis file is a part of the Multi-Worm Tracker and is distributed under the\nterms of the GNU Lesser General Public Licence version 2.1 (LGPL 2.1).\nFor details, see GPL2.txt and LGPL2.1.txt, or http://www.gnu.org/licences\n \nTo contact the authors, email kerrlab@users.sourceforge.net."
  # "Device Start Timing Control"
  # "Main Controls Cluster"
  # "Assorted buttons for advanced settings/ROI/reference objects"
  # "Stimulus Timing Controls"
  # "Exp. Duration"
  # "Array of ROIs"
  # "Statistics data controls"
  # "Display Controls; \ndisplay type and display on/off toggle"
  # "Settigns-related buttons"
  # "ROI-related buttons"
  # "Reference Object-related buttons"
  # "Overall control buttons"
  # "Image Bit Depth Control"
  # "Function Generator Settings"
  # "Image/Tracking Parameters"
  # "Blob Tracking Parameters"
  # "State variables"
  # "Images"
  # "Hardware System names/handles"
  # "Graph FP objects and controls"
  # "Stimulus delivery control parameters"
  # "Stimulus control signal parameters"
  # "Front panel indicators"
  # "Data output parameters"
  # "References to the front panel controls"
  n1 = control-ref of="AFG resource name"() -> (w70:refnum<vi>)
  n2 = control-ref of="Turn on Background division algorithm"() -> (w4:refnum<vi>)
  n3 = control-ref of="Turn on external triggering of camera"() -> (w2:refnum<vi>)
  n4 = control-ref of="Turn on output aggregation?"() -> (w5:refnum<vi>)
  n5 = control-ref of="Run"() -> (w101:refnum<vi>)
  n6 = control-ref of="Save"() -> (w16:refnum<vi>)
  n7 = control-ref of="Load"() -> (w17:refnum<vi>)
  n8 = control-ref of="Set Region of Interest"() -> (w115:refnum<vi>)
  n9 = control-ref of="Clear Region of Interest"() -> (w118:refnum<vi>)
  n10 = control-ref of="Clear Reference Object(s)"() -> (w117:refnum<vi>)
  n11 = control-ref of="Set New Reference Object"() -> (w116:refnum<vi>)
  n12 = control-ref of="Advanced Settings"() -> (w87:refnum<vi>)
  n13 = control-ref of="Custom 2"() -> (w8:refnum<vi>)
  n14 = control-ref of="Advanced Custom 2 Settings"() -> (w13:refnum<vi>)
  n15 = control-ref of="Tap"() -> (w49:refnum<vi>)
  n16 = control-ref of="Advanced Tap Settings"() -> (w44:refnum<vi>)
  n17 = control-ref of="Puff"() -> (w43:refnum<vi>)
  n18 = control-ref of="Advanced Puff Settings"() -> (w38:refnum<vi>)
  n19 = control-ref of="Custom 1"() -> (w37:refnum<vi>)
  n20 = control-ref of="Advanced Custom 1 Settings"() -> (w32:refnum<vi>)
  n21 = control-ref of="Type of object to track"() -> (w84:refnum<vi>)
  n22 = control-ref of="Contour?"() -> (w77:refnum<vi>)
  n23 = control-ref of="Skeletonize?"() -> (w76:refnum<vi>)
  n24 = control-ref of="Bit Depth from Camera?"() -> (w71:refnum<vi>)
  n25 = control-ref of="Raw Image Save Interval (s)"() -> (w7:refnum<vi>)
  n26 = control-ref of="Custom 2"() -> (w19:refnum<vi>)
  n27 = control-ref of="Custom 2 Delay"() -> (w9:refnum<vi>)
  n28 = control-ref of="Custom 2 Interval"() -> (w10:refnum<vi>)
  n29 = control-ref of="Custom 2 Number"() -> (w11:refnum<vi>)
  n30 = control-ref of="Custom 1"() -> (w92:refnum<vi>)
  n31 = control-ref of="Auto-start delay (s)"() -> (w52:refnum<vi>)
  n32 = control-ref of="Number of Image Adaptation Bands"() -> (w51:refnum<vi>)
  n33 = control-ref of="Experiment Duration (s)"() -> (w50:refnum<vi>)
  n34 = control-ref of="Tap Delay"() -> (w48:refnum<vi>)
  n35 = control-ref of="Tap Interval"() -> (w47:refnum<vi>)
  n36 = control-ref of="Tap Number"() -> (w46:refnum<vi>)
  n37 = control-ref of="Puff Delay"() -> (w42:refnum<vi>)
  n38 = control-ref of="Puff Interval"() -> (w41:refnum<vi>)
  n39 = control-ref of="Puff Number"() -> (w40:refnum<vi>)
  n40 = control-ref of="Custom 1 Delay"() -> (w36:refnum<vi>)
  n41 = control-ref of="Custom 1 Interval"() -> (w35:refnum<vi>)
  n42 = control-ref of="Custom 1 Number"() -> (w34:refnum<vi>)
  n43 = control-ref of="Object Contrast (%)"() -> (w83:refnum<vi>)
  n44 = control-ref of="Fill Hysteresis (%)"() -> (w82:refnum<vi>)
  n45 = control-ref of="Maximum Object Size (pixels)"() -> (w81:refnum<vi>)
  n46 = control-ref of="Minimum Object Size (pixels)"() -> (w80:refnum<vi>)
  n47 = control-ref of="Object Size hysteresis (%)"() -> (w79:refnum<vi>)
  n48 = control-ref of="Frames of Adaptation"() -> (w75:refnum<vi>)
  n49 = control-ref of="Adaptation Rate"() -> (w74:refnum<vi>)
  n50 = control-ref of="Object Border"() -> (w73:refnum<vi>)
  n51 = control-ref of="Image Bit Depth"() -> (w72:refnum<vi>)
  n52 = control-ref of="Puff"() -> (w109:refnum<vi>)
  n53 = control-ref of="custom 2 fraction of time between is active"() -> (w14:refnum<vi>)
  n54 = control-ref of="time between custom 2 onset"() -> (w15:refnum<vi>)
  n55 = control-ref of="Prefix"() -> (w85:refnum<vi>)
  n56 = control-ref of="IMAQ Camera Interface Name"() -> (w69:refnum<vi>)
  n57 = control-ref of="puff fraction of time between is active"() -> (w31:refnum<vi>)
  n58 = control-ref of="time between puff onset"() -> (w30:refnum<vi>)
  n59 = control-ref of="tap fraction of time between is active"() -> (w29:refnum<vi>)
  n60 = control-ref of="time between tap onset"() -> (w28:refnum<vi>)
  n61 = control-ref of="Tap Train Number"() -> (w27:refnum<vi>)
  n62 = control-ref of="custom 1 fraction of time between is active"() -> (w26:refnum<vi>)
  n63 = control-ref of="time between custom 1 onset"() -> (w25:refnum<vi>)
  n64 = control-ref of="Custom 2 Interval"() -> (w21:refnum<vi>)
  n65 = control-ref of="Custom 2 Number"() -> (w22:refnum<vi>)
  n66 = control-ref of="Custom 1 Interval"() -> (w90:refnum<vi>)
  n67 = control-ref of="Custom 1 Number"() -> (w89:refnum<vi>)
  n68 = control-ref of="Custom 2 Delay"() -> (w20:refnum<vi>)
  n69 = control-ref of="Custom 2 Stimulus Method"() -> (w12:refnum<vi>)
  n70 = control-ref of="Tap"() -> (w113:refnum<vi>)
  n71 = control-ref of="Custom 1 Delay"() -> (w91:refnum<vi>)
  n72 = control-ref of="Path"() -> (w86:refnum<vi>)
  n73 = control-ref of="Tap Stimulus Method"() -> (w45:refnum<vi>)
  n74 = control-ref of="Puff Stimulus Method"() -> (w39:refnum<vi>)
  n75 = control-ref of="Custom 1 Stimulus Method"() -> (w33:refnum<vi>)
  n76 = control-ref of="Image Binning"() -> (w78:refnum<vi>)
  n77 = control-ref of="Puff Delay"() -> (w108:refnum<vi>)
  n78 = control-ref of="Puff Interval"() -> (w107:refnum<vi>)
  n79 = control-ref of="Puff Number"() -> (w106:refnum<vi>)
  n80 = control-ref of="Custom 2 Stimulus Method"() -> (w23:refnum<vi>)
  n81 = control-ref of="Tap Delay"() -> (w112:refnum<vi>)
  n82 = control-ref of="Tap Interval"() -> (w111:refnum<vi>)
  n83 = control-ref of="Tap Number"() -> (w110:refnum<vi>)
  n84 = control-ref of="Custom 1 Stimulus Method"() -> (w88:refnum<vi>)
  n85 = control-ref of="Puff Stimulus Method"() -> (w104:refnum<vi>)
  n86 = control-ref of="Tap Stimulus Method"() -> (w105:refnum<vi>)
  n87 = Bundle("Puff"=w109, "Puff Delay"=w108, "Puff Interval"=w107, "Puff Number"=w106, "Puff Stimulus Method"=w104) -> (w102:T4)  [unwired: 1 in]
  n88 = Bundle("Custom 2"=w19, "Custom 2 Delay"=w20, "Custom 2 Interval"=w21, "Custom 2 Number"=w22, "Custom 2 Stimulus Method"=w23) -> (w18:T5)  [unwired: 1 in]
  n89 = Bundle("Custom 1"=w92, "Custom 1 Delay"=w91, "Custom 1 Interval"=w90, "Custom 1 Number"=w89, "Custom 1 Stimulus Method"=w88) -> (w93:T6)  [unwired: 1 in]
  n90 = Bundle("Tap"=w113, "Tap Delay"=w112, "Tap Interval"=w111, "Tap Number"=w110, "Tap Stimulus Method"=w105) -> (w103:T7)  [unwired: 1 in]
  n91 = Bundle(w103, w102, w93, w18) -> (w6:T8)  [unwired: 1 in]
  n92 = Bundle("Run"=w101, "Set Region of Interest"=w115, "Clear Region of Interest"=w118, "Clear Reference Object(s)"=w117, "Set New Reference Object"=w116, "Advanced Settings"=w87) -> (w97:T9)  [unwired: 1 in]
  n93 = Bundle("Path"=w86, "Prefix"=w85, "Type of object to track"=w84, "Object Contrast (%)"=w83, "Fill Hysteresis (%)"=w82, "Maximum Object Size (pixels)"=w81, "Minimum Object Size (pixels)"=w80, "Object Size hysteresis (%)"=w79, "Image Binning"=w78, "Contour?"=w77, "Skeletonize?"=w76, "Frames of Adaptation"=w75, "Adaptation Rate"=w74, "Object Border"=w73, "Image Bit Depth"=w72, "Bit Depth from Camera?"=w71, "AFG resource name"=w70, "IMAQ Camera Interface Name"=w69, "Auto-start delay (s)"=w52, "Number of Image Adaptation Bands"=w51, "Experiment Duration (s)"=w50, "Tap"=w49, "Tap Delay"=w48, "Tap Interval"=w47, "Tap Number"=w46, "Tap Stimulus Method"=w45, "Advanced Tap Settings"=w44, "Puff"=w43, "Puff Delay"=w42, "Puff Interval"=w41, "Puff Number"=w40, "Puff Stimulus Method"=w39, "Advanced Puff Settings"=w38, "Custom 1"=w37, "Custom 1 Delay"=w36, "Custom 1 Interval"=w35, "Custom 1 Number"=w34, "Custom 1 Stimulus Method"=w33, "Advanced Custom 1 Settings"=w32, "puff fraction of time between is active"=w31, "time between puff onset"=w30, "tap fraction of time between is active"=w29, "time between tap onset"=w28, "Tap Train Number"=w27, "custom 1 fraction of time between is active"=w26, "time between custom 1 onset"=w25, "Custom 2"=w8, "Custom 2 Delay"=w9, "Custom 2 Interval"=w10, "Custom 2 Number"=w11, "Custom 2 Stimulus Method"=w12, "Advanced Custom 2 Settings"=w13, "custom 2 fraction of time between is active"=w14, "time between custom 2 onset"=w15, "Save"=w16, "Load"=w17, "Raw Image Save Interval (s)"=w7, "Turn on output aggregation?"=w5, "Turn on Background division algorithm"=w4, "Turn on external triggering of camera"=w2) -> (w98:T10)  [unwired: 1 in]
  n94 = Cluster To Array(cluster=w97) -> (array=w114:refnum<vi>[])
  n95 = call "make_buttons_available.vi"("array"=w114, "Make Available"=TRUE) -> ()
  n96 = call "make_controls_available.vi"("input cluster"=w98, "Make Available"=TRUE) -> ()
  n97 = Bundle(w6, w98, w97) -> (w96:T11)  [unwired: 1 in]
  n98 = flat-sequence {
    tunnel: [w121] -> w64
    tunnel: [w119] -> w63
    tunnel: w96 -> [w121]
    tunnel: [w205] -> w95
    tunnel: w64 -> [w205]
    tunnel: w63 -> [w193]
    tunnel: [w193] -> w62
    tunnel: w95 -> [w222]
    tunnel: [w222] -> w58
    tunnel: [w232] -> w56
    tunnel: w62 -> [w227]
    tunnel: [w226] -> w54
    tunnel: w58 -> [w371]
    tunnel: [w371] -> w57
    tunnel: w56 -> [w370]
    tunnel: [w370] -> w55
    tunnel: w54 -> [w369]
    tunnel: [w369] -> w53
    tunnel: w57 -> [w425]
    tunnel: [w384] -> w94
    tunnel: w55 -> [w384]
    tunnel: [w425] -> w67
    tunnel: w53 -> [w419]
    tunnel: [w414] -> w61
    tunnel: [w391] -> w59
    tunnel: w94 -> [w496]
    tunnel: [w469] -> w68
    tunnel: w67 -> [w469]
    tunnel: w61 -> [w462]
    tunnel: [w466] -> w60
    tunnel: w59 -> [w465]
    tunnel: w68 -> [w776]
    tunnel: w60 -> [w774]
    frame #0 {
      n99 = property on="Query for Interface?" class="Bool (strict)"() -> ("Value"=w120:bool)  [unwired: 2 in, 2 out]
      n100 = case shown="True" w120 {
        tunnel: [w123 w150] -> w119
        frame False {
          n101 = property on="Image Data Input Source" class="Enum (strict)"() -> ("Value"=w125:T1)  [unwired: 2 in, 2 out]
          n102 = case shown="\"AVI file\"" w125 {
            tunnel: [_ w137 _] -> w124
            tunnel: [w133 _ _] -> w127
            tunnel: [_ _ w146] -> w126
            frame "IMAQ interface", Default {
              n103 = property on="IMAQ Camera Interface Name" class="Str"() -> ("Value"=w130:string)  [unwired: 2 in, 2 out]
              n104 = call <vilib>:"IMAQ Init.vi"("Interface Name"=w130) -> ("error out"=w132:errorcluster, "IMAQ Session Out"=w131:refnum<k11>)  [unwired: 9 in]
              n105 = call <vilib>:"IMAQ Grab Setup.vi"("error in (no error)"=w132, "IMAQ Session In"=w131) -> ("error out"=w129:errorcluster, "IMAQ Session Out"=w133:refnum<k11>)  [unwired: 8 in]
              n106 = Unbundle(w129) -> ("status"=w128:bool)  [unwired: 2 out]
              n107 = case shown="True" w128 {
                frame False {
                }
                frame True {
                  n108 = flat-sequence {
                    frame #0 {
                      n109 = call "Display Message to User3"() -> ()  [unwired: 10 in, 2 out]
                    }
                    frame #1 {
                      n110 = property on="Query for Interface?" class="Bool (strict)"("Value"=TRUE ("Query for Interface?")) -> ()  [unwired: 2 in, 2 out]
                    }
                    frame #2 {
                      n111 = Stop(stop? (T)=TRUE) -> ()
                    }
                  }
                }
              }
            }
            frame "IMAQdx interface" {
              n112 = property on="IMAQdx camera interface name" class="IMAQdx (strict)"() -> ("Value"=w138:refnum<k21>)  [unwired: 2 in, 2 out]
              n113 = call <vilib>:"IMAQdx Open Camera.vi"("Session In"=w138) -> ("error out"=w140:errorcluster, "Session Out"=w139:T2)  [unwired: 9 in]
              n114 = call <vilib>:"IMAQdx Configure Grab.vi"("error in"=w140, "Session In"=w139) -> ("error out"=w136:errorcluster, "Session Out"=w137:T2)  [unwired: 8 in]
              n115 = Unbundle(w136) -> ("status"=w141:bool)  [unwired: 2 out]
              n116 = case shown="True" w141 {
                frame False {
                }
                frame True {
                  n117 = flat-sequence {
                    frame #0 {
                      n118 = call "Display Message to User4"() -> ()  [unwired: 10 in, 2 out]
                    }
                    frame #1 {
                      n119 = property on="Query for Interface?" class="Bool (strict)"("Value"=TRUE ("Query for Interface?")) -> ()  [unwired: 2 in, 2 out]
                    }
                    frame #2 {
                      n120 = Stop(stop? (T)=TRUE) -> ()
                    }
                  }
                }
              }
            }
            frame "AVI file" {
              n121 = property on="AVI path" class="Path"() -> ("Value"=w147:path)  [unwired: 2 in, 2 out]
              n122 = call "IMAQ AVI Open"("AVI Path"=w147) -> ("error out"=w144:errorcluster, "Avi Refnum"=w146:T13)  [unwired: 9 in]
              n123 = Unbundle(w144) -> ("status"=w145:bool)  [unwired: 2 out]
              n124 = case shown="True" w145 {
                frame False {
                }
                frame True {
                  n125 = flat-sequence {
                    frame #0 {
                      n126 = call "Display Message to User5"() -> ()  [unwired: 10 in, 2 out]
                    }
                    frame #1 {
                      n127 = property on="Query for Interface?" class="Bool (strict)"("Value"=TRUE ("Query for Interface?")) -> ()  [unwired: 2 in, 2 out]
                    }
                    frame #2 {
                      n128 = Stop(stop? (T)=TRUE) -> ()
                    }
                  }
                }
              }
            }
          }
          n129 = property on="Turn on external triggering of camera" class="Bool (strict)"() -> ("Value"=w122:bool)  [unwired: 2 in, 2 out]
          n130 = Bundle("IMAQ Session Out"=w127, "Avi Refnum"=w126, "Value"=w125, "Session Out"=w124, "Value"=w122) -> (w123:T14)  [unwired: 1 in]
        }
        frame True {
          n131 = flat-sequence {
            tunnel: [w161] -> w157
            tunnel: [w167] -> w155
            tunnel: [w166] -> w153
            tunnel: [w165] -> w152
            tunnel: w157 -> [w173]
            tunnel: [w173] -> w156
            tunnel: w155 -> [w172]
            tunnel: [w172] -> w154
            tunnel: w153 -> [w171]
            tunnel: w152 -> [w170]
            tunnel: [w169] -> w151
            tunnel: w156 -> [w187]
            tunnel: w154 -> [_]
            tunnel: w151 -> [w186]
            tunnel: [w185] -> w150
            frame #0 {
              n132 = property on="IMAQ Camera Interface Name" class="Str"() -> ("Value"=w168:string)  [unwired: 2 in, 2 out]
              n133 = property on="Turn on external triggering of camera" class="Bool (strict)"() -> ("Value"=w159:bool)  [unwired: 2 in, 2 out]
              n134 = call "camera_selector.vi"("IMAQ interface name"=w168, "Use external trigger for camera control (IMAQ only)"=w159) -> ("image acq settings"=w167:T15)
              n135 = Unbundle(w167) -> ("IMAQ Session"=w164:refnum<k11>, "AVI Refnum"=w163:refnum<k1>, "Image Data Input Source"=w162:T16, w161:T17, "error?"=w166:bool, "use extrenal trigger"=w160:bool, "SR handle"=w158:u32)
              n136 = Bundle("IMAQ Session"=w164, "AVI Refnum"=w163, "Image Data Input Source"=w162, "SR handle"=w158) -> (w165:T18)  [unwired: 1 in]
              n137 = property on="Turn on external triggering of camera" class="Bool (strict)"("Value"=w160) -> ()  [unwired: 2 in, 2 out]
            }
            frame #1 {
              n138 = case shown="False" w171 {
                tunnel: w170 -> [w174 _]
                tunnel: [w174 _] -> w169
                frame False {
                }
                frame True {
                  n139 = flat-sequence {
                    frame #0 {
                      n140 = call "Display Message to User2"() -> ()  [unwired: 10 in, 2 out]
                    }
                    frame #1 {
                      n141 = property on="Query for Interface?" class="Bool (strict)"("Value"=TRUE ("Query for Interface?")) -> ()  [unwired: 2 in, 2 out]
                    }
                    frame #2 {
                      n142 = Stop(stop? (T)=TRUE) -> ()
                    }
                  }
                }
              }
            }
            frame #2 {
              n143 = Unbundle(w187) -> ("IMAQ Name"=w188:string, "IMAQDx Session"=w180:T2, "AVI/MMF Path"=w179:path)
              n144 = Unbundle(w186) -> ("IMAQ Session"=w184:refnum<k11>, "AVI Refnum"=w183:refnum<k1>, "Image Data Input Source"=w181:T16, "SR handle"=w177:u32)
              n145 = property on="IMAQ Camera Interface Name" class="Str"("Value"=w188) -> ()  [unwired: 2 in, 2 out]
              n146 = property on="IMAQdx camera interface name" class="IMAQdx (strict)"("Value"=w180) -> ()  [unwired: 2 in, 2 out]
              n147 = property on="AVI path" class="Path"("Value"=w179) -> ()  [unwired: 2 in, 2 out]
              n148 = property on="Turn on external triggering of camera" class="Bool (strict)"() -> ("Value"=w178:bool)  [unwired: 2 in, 2 out]
              n149 = Bundle("IMAQ Session"=w184, "AVI Refnum"=w183, "Image Data Input Source"=w181, "IMAQDx Session"=w180, "Value"=w178, "SR handle"=w177) -> (w185:T19)  [unwired: 1 in]
              n150 = property on="Query for Interface?" class="Bool (strict)"("Value"=FALSE ("Query for Interface?")) -> ()  [unwired: 2 in, 2 out]
              n151 = property on="Image Data Input Source" class="Enum (strict)"("Value"=w181) -> ()  [unwired: 2 in, 2 out]
            }
          }
        }
      }
    }
    frame #1 {
      w206 = T20 1 items=["Grayscale (U8)", "Grayscale (I16)", "Grayscale (SGL)", "Complex (CSG)", "RGB (U32)", "HSL (U32)", "RGB (U64)"] ("Image Type")
      # "MWT_getNewHandle"
      # "Create memory for displayed image"
      # "Dis/enable run button"
      # "Set initial state of important buttons"
      # "Stimulus Delivery Setup"
      # "Initial Set up"
      n152 = call "Init_Stimulus.vi"() -> ()  [unwired: 1 in]
      n153 = property on="Stop" class="Bool (strict)"("Disabled"=u8 0, "Value"=FALSE) -> ()  [unwired: 2 in, 2 out]
      n154 = property on="Run" class="Bool (strict)"("Value"=FALSE) -> ()  [unwired: 2 in, 2 out]
      n155 = property on="Display/Don't Display" class="Bool (strict)"("Value"=TRUE) -> ()  [unwired: 2 in, 2 out]
      n156 = Unbundle(w205) -> (w191:T10)  [unwired: 2 out]
      n157 = property on="last acquired buffer" class="DigNum (strict)"("Value"=0 ("last acquired buffer")) -> ()  [unwired: 2 in, 2 out]
      n158 = local read "ROI Array"() -> (w212:dbl[][])
      n159 = call "init_ROI.vi"("Input ROI Array"=w212, "camera cluster"=w193) -> ("First Call? out"=w210:bool, "Output ROI Array"=w211:dbl[][])
      n160 = dll-call lib="C:/Users/Marc/multi worm tracker/MWT_1.3.0_r1035/MultiWorm Tracker v1.3.0/data/MWT.dll" fn="MWT_getNewHandle"() -> ("return type"=w190:i32)  [unwired: 3 in, 2 out]
      "Tracker Handle" <- w190
      n161 = local write "First-call"(w210) -> ()
      n162 = call "set_in_library.vi"("Cluster"=w191, "camera cluster"=w193, "Tracker Handle"=w190, "Array"=w211) -> ("Directory Exists?"=w199:bool)  [unwired: 1 out]
      n163 = call "BitsPerPixel.vi"("camera cluster"=w193) -> ("BitsPerPixel"=w196:u32)
      n164 = call "GetWidthAndHeight.vi"(0:w193) -> ("Width"=w195:u32, "Height"=w194:u32)
      n165 = local write "ROI Array"(w211) -> ()
      n166 = control-ref of="Directory Exists?"() -> (w198:refnum<vi>)
      n167 = call "IMAQ Create"("Image Name"="image data", "Image Type"=w206) -> ("New Image"=w209:T3, "error out"=w189:errorcluster)  [unwired: 3 in]
      n168 = Greater?(x=w196, y=u32 8) -> (0:w203:bool)
      n169 = Select(t=0, s=w199, f=2) -> (s? t:f=w200:i32)
      n170 = property on="Run" class="Bool (strict)"("Disabled"=w200) -> ()  [unwired: 2 in, 2 out]
      n171 = case shown="True" FALSE {
        tunnel: w203 -> [_ w217]
        frame False {
        }
        frame True {
          n172 = case shown="False" w217 {
            frame False {
              n173 = call "Display Message to User"() -> ()  [unwired: 10 in, 2 out]
            }
            frame True {
              # "Everything\nis fine."
            }
          }
        }
      }
      n174 = property class="Bool (strict)"(reference=w198, "Value"=w199) -> ()  [unwired: 1 in, 2 out]
      n175 = call "IMAQ SetImageSize"("error in (no error)"=w189, "Y Resolution"=w194, "X Resolution"=w195, "Image"=w209) -> ("Image Out"=w208:T3)  [unwired: 1 in, 1 out]
      n176 = property on="Image" class="ImageControl"("Value"=w208) -> ()  [unwired: 2 in, 2 out]
    }
    frame #2 {
      # "Initial feedback and settings configuration"
      # "Initial Constants with dummy values"
      n177 = local read "custom 1 timing array"() -> (w220:dbl[])
      n178 = local read "custom 2 timing array"() -> (w221:dbl[])
      n179 = local read "puff timing array"() -> (w219:dbl[])
      n180 = local read "tap timing array"() -> (w218:dbl[])
      n181 = local read "AFG resource name"() -> (w228:refnum<k15>)
      n182 = Unbundle(w222) -> (w223:T10)  [unwired: 2 out]
      n183 = call "get_tracker_settings.vi"("Cluster"=w223) -> ("settings value cluster"=w235:T21)
      n184 = while {
        shift-right: [w245] -> w233
        shift-left: w218 -> [w308]
        shift-right: [w311] -> _
        shift-left: T12 {"Value"=FALSE, "Value"=-1000.0, "Value"=-1000.0, "Value"=1000, "Value"=1000} ("output values cluster") -> [w278]
        shift-right: [w252] -> _
        shift-left: w235 -> [w314]
        shift-right: [w305] -> _
        shift-left: T12 {"Value"=FALSE, "Value"=-1000.0, "Value"=-1000.0, "Value"=1000, "Value"=1000} ("output values cluster") -> [w277]
        shift-right: [w244] -> w234
        shift-left: w219 -> [w307]
        shift-right: [w317] -> _
        shift-left: w228 -> [w318]
        tunnel: w222 -> [w299]
        shift-right: [w243] -> w230
        shift-left: w220 -> [w306]
        shift-right: [w304] -> _
        shift-left: T12 {"Value"=FALSE, "Value"=-1000.0, "Value"=-1000.0, "Value"=1000, "Value"=1000} ("output values cluster") -> [w276]
        shift-right: [w301] -> _
        shift-left: TRUE -> [w300]
        tunnel: w227 -> [w266]
        tunnel: [w266] -> w226
        shift-right: [w273] -> _
        shift-left: T12 {"Value"=FALSE, "Value"=-1000.0, "Value"=-1000.0, "Value"=1000, "Value"=1000} ("output values cluster") -> [w275]
        shift-right: [w242] -> w224
        shift-left: w221 -> [w274]
        stop <- w284 stop-if-true
        # "Note: Condition necessary\nbecause of potential discrepency\nbetween closing camera sessions\nand exiting the VI."
        # "Logic for \"begin after ... seconds\" function"
        # "Dis/enable run button"
        # "Feedback on setup stage"
        # "UI for ROIs"
        # "UI for advanced settings"
        # "AFG initialization"
        # "UI for reference objects"
        # "Sets values in library,\nas well as saving and loading"
        # "Sets up the timing arrays \nfor the stimuli"
        # "Clean-up if stop is pressed."
        n185 = Unbundle(w299) -> (w279:T8, w268:T10)  [unwired: 1 out]
        n186 = local read "AFG resource name"() -> (w319:refnum<k15>)
        n187 = Unbundle(w299) -> (w267:T9)  [unwired: 2 out]
        n188 = property on="User interface display slector" class="Ring (strict)"() -> ("Value"=w241:u16)  [unwired: 2 in, 2 out]
        n189 = case shown="0, Default" w241 {
          frame 0, Default {
            w321 = u16 0 items=["Raw Image", "Memory Image", "Fixed Image"] ("What to display")
            n190 = property on="Display/Don't Display" class="Bool (strict)"("Value"=TRUE ("Display/Don't Display")) -> ()  [unwired: 2 in, 2 out]
            n191 = property on="What to display" class="Ring (strict)"("Value"=w321) -> ()  [unwired: 2 in, 2 out]
          }
          frame 1 {
            w323 = u16 1 items=["Raw Image", "Memory Image", "Fixed Image"] ("What to display")
            n192 = property on="Display/Don't Display" class="Bool (strict)"("Value"=TRUE ("Display/Don't Display")) -> ()  [unwired: 2 in, 2 out]
            n193 = property on="What to display" class="Ring (strict)"("Value"=w323) -> ()  [unwired: 2 in, 2 out]
          }
          frame 2 {
            w325 = u16 2 items=["Raw Image", "Memory Image", "Fixed Image"] ("What to display")
            n194 = property on="Display/Don't Display" class="Bool (strict)"("Value"=TRUE ("Display/Don't Display")) -> ()  [unwired: 2 in, 2 out]
            n195 = property on="What to display" class="Ring (strict)"("Value"=w325) -> ()  [unwired: 2 in, 2 out]
          }
          frame 3 {
            w327 = u16 2 items=["Raw Image", "Memory Image", "Fixed Image"] ("What to display")
            n196 = property on="Display/Don't Display" class="Bool (strict)"("Value"=FALSE ("Display/Don't Display")) -> ()  [unwired: 2 in, 2 out]
            n197 = property on="What to display" class="Ring (strict)"("Value"=w327) -> ()  [unwired: 2 in, 2 out]
          }
        }
        n198 = local read "AFG Settings"() -> (w309:dbl[][])
        n199 = local read "Image Bit Depth"() -> (w262:u32)
        n200 = property on="Tracker Handle" class="DigNum (strict)"() -> ("Value"=w316:i32)  [unwired: 2 in, 2 out]
        n201 = property on="last acquired buffer" class="DigNum (strict)"() -> ("Value"=w290:i32)  [unwired: 2 in, 2 out]
        n202 = Not Equal?(x=w319, y=w318) -> (x != y?=w303:bool)
        n203 = And(x=w303, y=w300) -> (x .and. y?=w302:bool)
        n204 = Bundle("AFG Settings"=w309, "tap timing array"=w308, "puff timing array"=w307, "custom timing array"=w306, "custom 2 timing array"=w274, w279, w268, "output values cluster"=w278, "output values cluster"=w277, "output values cluster"=w276, "output values cluster"=w275) -> (w310:T22)  [unwired: 1 in]
        n205 = Bundle(w266, "Value"=w316, "Value"=w290) -> (w313:T23)  [unwired: 1 in]
        n206 = case shown="True" w302 {
          tunnel: [w340 w343] -> w317
          tunnel: w319 -> [_ w343]
          tunnel: w318 -> [w340 _]
          tunnel: [w339 FALSE] -> w301
          tunnel: w300 -> [w339 _]
          frame False {
          }
          frame True {
            n207 = call "AFG_Init.vi"("amplitude (1)"=1.0, "resource name"=w343, "frequency (1000000)"=100.0) -> ("instrument handle out"=w341:refnum<k15>)
            n208 = local write "AFG instrument handle"(w341) -> ()
          }
        }
        n209 = call "all_things_stimulus.vi"("input cluster"=w310) -> ("output cluster"=w312:T24)
        n210 = Bundle(w313, w267, "Image Bit Depth"=w262) -> (w240:T25)  [unwired: 1 in]
        n211 = Unbundle(w312) -> ("output values cluster"=w311:T26, "Output Array"=w249:dbl[], "output values cluster"=w305:T26, "Output Array"=w248:dbl[], "output values cluster"=w304:T26, "Output Array"=w247:dbl[], "AFG Settings"=w254:dbl[][], "output values cluster"=w273:T26, "Output Array"=w246:dbl[])
        n212 = call "set_or_clear_reference_object.vi"("input cluster"=w240) -> ("last acquired buffer out"=w292:i32)
        n213 = local read "ROI Array"() -> (w315:dbl[][])
        n214 = property on="last acquired buffer" class="DigNum (strict)"("Value"=w292) -> ()  [unwired: 2 in, 2 out]
        n215 = control-ref of="Directory Exists?"() -> (w253:refnum<vi>)
        n216 = Unbundle(w299) -> (w265:T10)  [unwired: 2 out]
        n217 = Bundle(w313, w268, "ROI Array"=w315, "settings value cluster"=w314, "AFG Settings"=w254, "Output Array"=w249, "Output Array"=w248, "Output Array"=w247, "Output Array"=w246) -> (w239:T27)  [unwired: 1 in]
        n218 = call "Tracker_Settings.vi"("input cluster"=w239, "Directory Exists?"=w253) -> ("output cluster"=w255:T28)
        n219 = Bundle(w265, w266) -> (w298:T29)  [unwired: 1 in]
        n220 = Unbundle(w255) -> ("Output  ROI Array"=w251:dbl[][], "settings value cluster"=w252:T21, "AFG Settings"=w250:dbl[][], "tap timing array"=w245:dbl[], "puff timing array"=w244:dbl[], "custom timing array"=w243:dbl[], "custom 2 timing array"=w242:dbl[])
        n221 = property on="last acquired buffer" class="DigNum (strict)"() -> ("Value"=w287:i32)  [unwired: 2 in, 2 out]
        n222 = property on="Tracker Handle" class="DigNum (strict)"() -> ("Value"=w286:i32)  [unwired: 2 in, 2 out]
        n223 = property on="Stop" class="Bool (strict)"() -> ("Value"=w269:bool)  [unwired: 2 in, 2 out]
        n224 = property on="Advanced Settings" class="Bool (strict)"() -> ("Value"=w297:bool)  [unwired: 2 in, 2 out]
        n225 = property on="Display/Don't Display" class="Bool (strict)"() -> ("Value"=w271:bool)  [unwired: 2 in, 2 out]
        n226 = Not(x=w269) -> (.not. x?=w272:bool)
        n227 = Bundle(w266, "Value"=w286, "Value"=w287) -> (w285:T23)  [unwired: 1 in]
        n228 = case shown="True" w297 {
          tunnel: w298 -> [_ w336]
          frame False {
          }
          frame True {
            n229 = call "advanced_settings.vi"("input cluster"=w336) -> ("Output AFG resource name"=w338:refnum<k15>)  [unwired: 1 out]
            n230 = local write "AFG resource name"(w338) -> ()
            n231 = property on="Advanced Settings" class="Bool (strict)"("Value"=FALSE ("Advanced Settings")) -> ()  [unwired: 2 in, 2 out]
          }
        }
        n232 = And(x=w271, y=w272) -> (x .and. y?=w270:bool)
        n233 = local write "AFG Settings"(w250) -> ()
        n234 = case shown="True" w270 {
          tunnel: w285 -> [_ w364]
          frame False {
          }
          frame True {
            n235 = local read "Image Binning"() -> (w363:u16)
            n236 = property on="What to display" class="Ring (strict)"() -> ("Value"=w359:u16)  [unwired: 2 in, 2 out]
            n237 = Bundle(w364, "Image Binning"=w363, "Value"=w359) -> (w352:T30)  [unwired: 1 in]
            n238 = call "initial_feedback.vi"("input cluster"=w352) -> ("output cluster"=w365:T31)
            n239 = Unbundle(w365) -> ("Acquired Buffer Number"=w362:i32, "return type"=w361:i32, "destination"=w360:i16[][])
            n240 = local read "Image Bit Depth"() -> (w354:u32)
            n241 = local read "Image"() -> (w366:T3)
            n242 = local write "Objects Found"(w361) -> ()
            n243 = property on="last acquired buffer" class="DigNum (strict)"("Value"=w362) -> ()  [unwired: 2 in, 2 out]
            n244 = call "IMAQ ArrayToImage"("Image Pixels (I16)"=w360, "Image"=w366) -> ("error out"=w353:errorcluster, "Image Out"=w358:T3)  [unwired: 8 in]
            n245 = call "IMAQ Image Bit Depth"("Image"=w358, "Bit Depth (0)"=w354, "error in (no error)"=w353, "Get/Set Bit Depth? (Set)"=TRUE) -> ("Image Out"=w357:T3, "error out"=→"error out":errorcluster)  [unwired: 9 in, 1 out]
            n246 = local write "Image"(w357) -> ()
          }
        }
        n247 = local write "ROI Array"(w251) -> ()
        n248 = local write "custom 2 timing array"(w242) -> ()
        n249 = local write "custom 1 timing array"(w243) -> ()
        n250 = local write "puff timing array"(w244) -> ()
        n251 = local write "tap timing array"(w245) -> ()
        n252 = local read "ROI Array"() -> (w259:dbl[][])
        n253 = Unbundle(w299) -> (w264:T10, w263:T9)  [unwired: 1 out]
        n254 = property on="First-call" class="Bool (strict)"() -> ("Value"=w260:bool)  [unwired: 2 in, 2 out]
        n255 = property on="Auto-start delay (s)" class="DigNum (strict)"() -> ("Value"=w281:i32)  [unwired: 2 in, 2 out]
        n256 = Greater Than 0?(x=w281) -> (x > 0?=w280:bool)
        n257 = control-ref of="Directory Exists?"() -> (w288:refnum<vi>)
        n258 = property on="last acquired buffer" class="DigNum (strict)"() -> ("Value"=w261:i32)  [unwired: 2 in, 2 out]
        n259 = property on="Tracker Handle" class="DigNum (strict)"() -> ("Value"=w289:i32)  [unwired: 2 in, 2 out]
        n260 = Bundle(w266, "Value"=w289, "Value"=w261) -> (w291:T23)  [unwired: 1 in]
        n261 = case shown="True" w280 {
          tunnel: [FALSE w335] -> w282
          frame False {
          }
          frame True {
            n262 = property on="Run" class="Bool (strict)"() -> ("Disabled"=w331:u8)  [unwired: 2 in, 2 out]
            n263 = Not Equal To 0?(x=w331) -> (x != 0?=w330:bool)
            n264 = property on="Auto-start delay (s)" class="DigNum (strict)"() -> ("Value"=w334:i32)  [unwired: 2 in, 2 out]
            n265 = call "Elapsed Time"("Time Target (s)"=w334, "Reset"=w330) -> ("Elapsed Time (s)"=w333:dbl, "Time has Elapsed"=w335:bool)  [unwired: 10 in, 6 out]
            n266 = Subtract(x=w334, y=w333) -> (x-y=w332:dbl)
            n267 = property on="Auto-start in (s)" class="DigNum (strict)"("Value"=w332) -> ()  [unwired: 2 in, 2 out]
          }
        }
        n268 = Bundle(w291, "ROI Array"=w259, "Value"=w260, w264, w263, "Directory Exists?"=w288) -> (w238:T32)  [unwired: 1 in]
        n269 = call "ROI.vi"("input cluster"=w238) -> ("Acquired Buffer Number"=w256:u32, "Output First-call"=w257:bool, "Output ROI Array"=w258:dbl[][])
        n270 = property on="Stop" class="Bool (strict)"() -> ("Value"=w320:bool)  [unwired: 2 in, 2 out]
        n271 = property on="First-call" class="Bool (strict)"("Value"=w257) -> ()  [unwired: 2 in, 2 out]
        n272 = local write "ROI Array"(w258) -> ()
        n273 = property on="last acquired buffer" class="DigNum (strict)"("Value"=w256) -> ()  [unwired: 2 in, 2 out]
        n274 = case shown="True" w320 {
          tunnel: w266 -> [_ w346]
          frame False {
          }
          frame True {
            n275 = flat-sequence {
              tunnel: w346 -> [w349]
              frame #0 {
                # "MWT_killHandle"
                n276 = property on="Tracker Handle" class="DigNum (strict)"() -> ("Value"=w348:i32)  [unwired: 2 in, 2 out]
                n277 = dll-call lib="C:/Users/Marc/multi worm tracker/MWT_1.3.0_r1035/MultiWorm Tracker v1.3.0/data/MWT.dll" fn="MWT_killHandle"("handle"=w348) -> ()  [unwired: 5 in, 2 out]
                n278 = Bundle(w349, 0) -> (w347:T33)  [unwired: 1 in]
                n279 = call "camera_closer.vi"("input cluster"=w347) -> ()
              }
              frame #1 {
                n280 = Stop(stop? (T)=TRUE) -> ()
              }
            }
          }
        }
        n281 = property on="Directory Exists?" class="Bool (strict)"() -> ("Value"=w293:bool)  [unwired: 2 in, 2 out]
        n282 = property on="Run" class="Bool (strict)"() -> ("Value"=w283:bool)  [unwired: 2 in, 2 out]
        n283 = Select(t=0, s=w293, f=2) -> (s? t:f=w294:i32)
        n284 = Or(x=w283, y=w282) -> (x .or. y?=w284:bool)
        n285 = property on="Run" class="Bool (strict)"("Disabled"=w294) -> ()  [unwired: 2 in, 2 out]
      }
      n286 = Bundle("tap timing array"=w233, "puff timing array"=w234, "custom timing array"=w230, "custom 2 timing array"=w224) -> (w232:T34)  [unwired: 1 in]
    }
    frame #3 {
      # "Special case for AVI input: Setting initial frame."
      n287 = Unbundle(w369) -> ("AVI Refnum"=w368:refnum<k1>, "Image Data Input Source"=w367:T16)  [unwired: 4 out]
      n288 = case shown="\"AVI file\"" w367 {
        tunnel: w368 -> [w376 _ _]
        frame "AVI file" {
          # "In the case of AVIs,\nreset the AVI frame\nto the \"beginning\" for\nprocessing."
          n289 = call "IMAQ AVI Get Info"("Avi Refnum"=w376) -> ("Frame Data"=w375:T35)  [unwired: 6 in, 4 out]
          n290 = Unbundle(w375) -> ("framesPerSecond"=w374:u32)  [unwired: 4 out]
          n291 = property on="Auto-start delay (s)" class="DigNum (strict)"() -> ("Value"=w373:i32)  [unwired: 2 in, 2 out]
          n292 = Multiply(x=w374, y=w373) -> (x*y=w372:u32)
          n293 = property on="last acquired buffer" class="DigNum (strict)"("Value"=w372) -> ()  [unwired: 2 in, 2 out]
        }
        frame "IMAQdx interface" {
          # "Do nothing for this interface"
        }
        frame "IMAQ interface" {
          # "Do nothing for this interface"
        }
      }
    }
    frame #4 {
      w377 = u16 3 items=["Raw Image", "Memory Image", "Fixed Image", "Nothing", ""] ("User interface display slector")
      w397 = 0
      w423 = FALSE ("Make Available")
      # "Configure initial settings of AFG."
      # "Output setup and disabling of controls"
      n294 = local read "AFG Settings"() -> (w394:dbl[][])
      n295 = property on="Image Binning" class="Ring (strict)"() -> ("Value"=w420:u16)  [unwired: 2 in, 2 out]
      n296 = property on="Frames of Adaptation" class="DigNum (strict)"() -> ("Value"=w421:i32)  [unwired: 2 in, 2 out]
      n297 = property on="User interface display slector" class="Ring (strict)"("Value"=w377) -> ()  [unwired: 2 in, 2 out]
      n298 = property on="Stop" class="Bool (strict)"("Disabled"=u8 0) -> ()  [unwired: 2 in, 2 out]
      n299 = property on="Display/Don't Display" class="Bool (strict)"("Value"=FALSE) -> ()  [unwired: 2 in, 2 out]
      n300 = Unbundle(w425) -> (w386:T10, w401:T9)  [unwired: 1 out]
      n301 = Index Array(array=w394, index (row) #1=w397, index (col) #1=1, index (row) #2=w397, index (col) #2=2) -> (element #1=w396:dbl, element #2=w395:dbl)
      n302 = local read "AFG instrument handle"() -> (w400:refnum<k15>)
      n303 = property on="Tracker Handle" class="DigNum (strict)"() -> ("Value"=w422:i32)  [unwired: 2 in, 2 out]
      n304 = property on="Prefix" class="Str"() -> ("Value"=w392:string)  [unwired: 2 in, 2 out]
      n305 = property on="last acquired buffer" class="DigNum (strict)"() -> ("Value"=w418:i32)  [unwired: 2 in, 2 out]
      n306 = local read "AFG Settings"() -> (w385:dbl[][])
      n307 = Concatenate Strings(w392, ".set") -> (w390:string)
      n308 = local read "Image"() -> (w413:T3)
      n309 = local read "ROI Array"() -> (w388:dbl[][])
      n310 = Cluster To Array(cluster=w401) -> (array=w424:refnum<vi>[])
      n311 = Bundle(w419, "Value"=w418) -> (w417:T36)  [unwired: 1 in]
      n312 = call "make_buttons_available.vi"("array"=w424, "Make Available"=w423) -> ()
      n313 = call "make_controls_available.vi"("input cluster"=w386, "Make Available"=w423) -> ()
      n314 = Unbundle(w417) -> (w416:T19)  [unwired: 1 out]
      n315 = Bundle(w417, "Value"=w422, "Value"=w421, "Value"=w420, "Image"=w413) -> (w379:T37)  [unwired: 1 in]
      n316 = call "AFG_Waveform_settings.vi"("amplitude (1)"=w395, "frequency (1000000)"=w396, "instrument handle"=w400) -> ()
      n317 = Unbundle(w384) -> ("tap timing array"=w382:dbl[], "puff timing array"=w383:dbl[], "custom timing array"=w381:dbl[], "custom 2 timing array"=w380:dbl[])
      n318 = call "set_date_and_create_initial_memory_image.vi"("input cluster"=w379) -> ("Acquired Buffer Number"=w405:u32, "sub_directory"=w402:string)
      n319 = property on="Path" class="Path"() -> ("Value"=w403:path)  [unwired: 2 in, 2 out]
      n320 = Bundle(w416, "Acquired Buffer Number"=w405) -> (w378:T38)  [unwired: 1 in]
      n321 = property on="Prefix" class="Str"() -> ("Value"=w407:string)  [unwired: 2 in, 2 out]
      n322 = Build Path(base path=w403, name or relative path=w402) -> (appended path=w391:path)
      n323 = Build Path(base path=w391, name or relative path=w390) -> (appended path=w387:path)
      n324 = Bundle(w386, "appended path"=w387, "ROI Array"=w388, "AFG Settings"=w385, "tap timing array"=w382, "puff timing array"=w383, "custom timing array"=w381, "custom 2 timing array"=w380) -> (w389:T39)  [unwired: 1 in]
      n325 = call "save_configuration.vi"("input cluster"=w389) -> ()
      n326 = Unbundle(w378) -> (w415:T19)  [unwired: 1 out]
      n327 = call "smart_get.vi"("Input Image"=w413, "Cluster"=w378) -> ("Image Out"=w412:T3, "Acquired Buffer Number"=w404:i32)
      n328 = Concatenate Strings(w407, ".png") -> (w410:string)
      n329 = Bundle(w415, "Acquired Buffer Number"=w404) -> (w414:T40)  [unwired: 1 in]
      n330 = Build Path(base path=w391, name or relative path=w410) -> (appended path=w409:path)
      n331 = property on="last acquired buffer" class="DigNum (strict)"("Value"=w404) -> ()  [unwired: 2 in, 2 out]
      n332 = call-poly "IMAQ Write File 2"("Use bit depth? (false)"=TRUE, "Image Quality"=u32 750, "File Path"=w409, "Image"=w412) -> ()  [unwired: 6 in, 2 out]
    }
    frame #5 {
      # "MWT_reportImageCorrectionAlgorithm"
      # "Individual Frame Saving and AFG control\nNOTE: These functions do not make sense when an AVI is used as input, and so are disabled in that case."
      # "Processing"
      n333 = Unbundle(w462) -> (w461:T19)  [unwired: 1 out]
      n334 = Unbundle(w461) -> ("Image Data Input Source"=w428:T16)  [unwired: 5 out]
      n335 = Not Equal?(x=w428, y=T1."AVI file" ("Image Data Input Source")) -> (x != y?=w463:bool)
      n336 = Unbundle(w496) -> ("tap timing array"=w435:dbl[], "puff timing array"=w433:dbl[], "custom timing array"=w431:dbl[], "custom 2 timing array"=w429:dbl[])
      n337 = case shown="True" w463 {
        tunnel: w465 -> [_ w523]
        tunnel: w462 -> [_ w520]
        frame False {
        }
        frame True {
          # "AFG control"
          n338 = local read "Image"() -> (w524:T3)
          n339 = property on="Raw Image Save Interval (s)" class="DigNum (strict)"() -> ("Value"=w519:dbl)  [unwired: 2 in, 2 out]
          n340 = call "IMAQ Create"("Image Name"="more_garbage") -> ("New Image"=w527:T3)  [unwired: 4 in, 1 out]
          n341 = Greater Than 0?(x=w519) -> (x > 0?=w525:bool)
          n342 = call "IMAQ Copy"("Image Dst"=w527, "Image Src"=w524) -> ("Image Dst Out"=w528:T3)  [unwired: 4 in, 1 out]
          n343 = Multiply(x=w519, y=1000.0) -> (x*y=w521:dbl)
          n344 = case shown="True" w525 {
            tunnel: w523 -> [_ w539]
            tunnel: w521 -> [_ w537]
            tunnel: w528 -> [_ w538]
            tunnel: w520 -> [_ w534]
            frame False {
            }
            frame True {
              n345 = call "get_time.vi"("input cluster"=w534) -> ("millisecond timer value"=w535:u32)
              n346 = while {
                tunnel: w539 -> [w557]
                tunnel: w537 -> [w550]
                tunnel: w538 -> [w556]
                tunnel: w534 -> [w541]
                shift-right: [w552] -> _
                shift-left: 0 -> [w551]
                shift-right: [w549] -> _
                shift-left: w535 -> [w554]
                tunnel: w535 -> [w548]
                stop <- w540 stop-if-true
                # "Larval-specific addition"
                n347 = Unbundle(w541) -> (w544:T19)  [unwired: 1 out]
                n348 = call "get_time.vi"("input cluster"=w541) -> ("millisecond timer value"=w549:u32)
                n349 = property on="last acquired buffer" class="DigNum (strict)"() -> ("Value"=w543:i32)  [unwired: 2 in, 2 out]
                n350 = Bundle(w544, "Value"=w543) -> (w542:T36)  [unwired: 1 in]
                n351 = Subtract(x=w549, y=w548) -> (x-y=w546:u32)
                n352 = call "elapsed_time.vi"("Time since last update"=w551, "Initial Time"=w554, "Current Time"=w549) -> ("Elapsed Time"=w547:i32)
                n353 = call "smart_get.vi"("Input Image"=w556, "Cluster"=w542) -> ("Image Out"=w555:T3, "Acquired Buffer Number"=w545:i32)
                n354 = Greater?(x=w547, y=w550) -> (0:w553:bool)
                n355 = property on="last acquired buffer" class="DigNum (strict)"("Value"=w545) -> ()  [unwired: 2 in, 2 out]
                n356 = case shown="True" w553 {
                  tunnel: w555 -> [_ w570]
                  tunnel: w557 -> [_ w569]
                  tunnel: [w558 0] -> w552
                  tunnel: w547 -> [w558 _]
                  tunnel: w546 -> [_ w559]
                  frame False {
                  }
                  frame True {
                    n357 = Format Into String(format string="%05d", w559) -> (resulting string=w566:string)  [unwired: 2 in, 1 out]
                    n358 = property on="Prefix" class="Str"() -> ("Value"=w567:string)  [unwired: 2 in, 2 out]
                    n359 = Concatenate Strings(w567, w566, ".png") -> (w564:string)
                    n360 = Build Path(base path=w569, name or relative path=w564) -> (appended path=w563:path)
                    n361 = call-poly "IMAQ Write File 2"("Use bit depth? (false)"=TRUE, "Image Quality"=u32 750, "File Path"=w563, "Image"=w570) -> ()  [unwired: 6 in, 2 out]
                  }
                }
                n362 = property on="Proccessing loop stopped?" class="Bool (strict)"() -> ("Value"=w540:bool)  [unwired: 2 in, 2 out]
              }
            }
          }
          n363 = local read "AFG Settings"() -> (w532:dbl[][])
          n364 = Array Size(array=w532) -> (size(s)=w533:i32[])
          n365 = call "get_time.vi"("input cluster"=w520) -> ("millisecond timer value"=w529:u32)
          n366 = Index Array(array=w533) -> (element=w530:i32)  [unwired: 1 in]
          n367 = while {
            tunnel: w532 -> [w579]
            shift-right: [w577] -> _
            shift-left: 0 -> [w578]
            tunnel: w530 -> [w581]
            tunnel: w529 -> [w580]
            tunnel: w520 -> [w572]
            stop <- w574 continue-if-true
            n368 = call "get_time.vi"("input cluster"=w572) -> ("millisecond timer value"=w576:u32)
            n369 = Less?(x=w578, y=w581) -> (x < y?=w575:bool)
            n370 = case shown="True" w575 {
              tunnel: w576 -> [_ w585]
              tunnel: w580 -> [_ w586]
              tunnel: w579 -> [_ w589]
              tunnel: w578 -> [w582 w588]
              tunnel: [w582 w587] -> w577
              frame False {
              }
              frame True {
                n371 = Index Array(array=w589, index (row) #1=w588, index (col) #1=0 ("disabled index (col)"), index (row) #2=w588, index (col) #2=1, index (row) #3=w588, index (col) #3=2) -> (element #1=w583:dbl, element #2=w594:dbl, element #3=w595:dbl)
                n372 = Subtract(x=w585, y=w586) -> (x-y=w584:u32)
                n373 = Greater Or Equal?(x=w584, y=w583) -> (x >= y?=w591:bool)
                n374 = case shown="True" w591 {
                  tunnel: w594 -> [_ w598]
                  tunnel: w595 -> [_ w597]
                  tunnel: w588 -> [w596 w601]
                  tunnel: [w596 w600] -> w587
                  frame False {
                  }
                  frame True {
                    n375 = local read "AFG instrument handle"() -> (w599:refnum<k15>)
                    n376 = Increment(x=w601) -> (x+1=w600:i32)
                    n377 = call "AFG_Waveform_settings.vi"("amplitude (1)"=w597, "frequency (1000000)"=w598, "instrument handle"=w599) -> ()
                  }
                }
              }
            }
            n378 = property on="Proccessing loop stopped?" class="Bool (strict)"() -> ("Value"=w571:bool)  [unwired: 2 in, 2 out]
            n379 = Not(x=w571) -> (.not. x?=w573:bool)
            n380 = And(x=w573, y=w575) -> (x .and. y?=w574:bool)
          }
        }
      }
      n381 = control-ref of="XY Graph"() -> (w482:refnum<vi>)
      n382 = control-ref of="XY Graph 2"() -> (w481:refnum<vi>)
      n383 = control-ref of="XY Graph 3"() -> (w480:refnum<vi>)
      n384 = control-ref of="XY Graph 4"() -> (w479:refnum<vi>)
      n385 = local read "Image"() -> (w497:T3)
      n386 = control-ref of="Graph Input"() -> (w486:refnum<vi>)
      n387 = control-ref of="Graph Input 2"() -> (w485:refnum<vi>)
      n388 = control-ref of="Graph Input 3"() -> (w484:refnum<vi>)
      n389 = control-ref of="Graph Input 4"() -> (w483:refnum<vi>)
      n390 = property on="tap fraction of time between is active" class="Arr (strict)"() -> ("Value"=w493:sgl[][])  [unwired: 2 in, 2 out]
      n391 = property on="time between tap onset" class="Arr (strict)"() -> ("Value"=w492:i32[][])  [unwired: 2 in, 2 out]
      n392 = property on="Tap Train Number" class="Arr (strict)"() -> ("Value"=w491:i32[][])  [unwired: 2 in, 2 out]
      n393 = call "IMAQ GetImageSize"("Image"=w497) -> ("Y Resolution"=w501:i32, "X Resolution"=w500:i32)  [unwired: 3 in, 1 out]
      n394 = property on="Image Binning" class="Ring (strict)"() -> ("Value"=w451:u16)  [unwired: 2 in, 2 out]
      n395 = Bundle("Graph Input"=w486, "Graph Input 2"=w485, "Graph Input 3"=w484, "Graph Input 4"=w483, "XY Graph"=w482, "XY Graph 2"=w481, "XY Graph 3"=w480, "XY Graph 4"=w479) -> (w478:T41)  [unwired: 1 in]
      n396 = property on="puff fraction of time between is active" class="Arr (strict)"() -> ("Value"=w489:sgl[][])  [unwired: 2 in, 2 out]
      n397 = property on="time between puff onset" class="Arr (strict)"() -> ("Value"=w488:i32[][])  [unwired: 2 in, 2 out]
      n398 = property on="Tracker Handle" class="DigNum (strict)"() -> ("Value"=w437:i32)  [unwired: 2 in, 2 out]
      n399 = property on="custom 2 fraction of time between is active" class="Arr (strict)"() -> ("Value"=w456:sgl[][])  [unwired: 2 in, 2 out]
      n400 = property on="time between custom 2 onset" class="Arr (strict)"() -> ("Value"=w455:i32[][])  [unwired: 2 in, 2 out]
      n401 = property on="custom 1 fraction of time between is active" class="Arr (strict)"() -> ("Value"=w476:sgl[][])  [unwired: 2 in, 2 out]
      n402 = property on="time between custom 1 onset" class="Arr (strict)"() -> ("Value"=w477:i32[][])  [unwired: 2 in, 2 out]
      n403 = call "get_time.vi"("input cluster"=w462) -> ("millisecond timer value"=w464:u32)
      n404 = Divide(x=w501, y=w451) -> (x/y=w505:dbl)
      n405 = Divide(x=w500, y=w451) -> (x/y=w506:dbl)
      n406 = dll-call lib="C:/Users/Marc/multi worm tracker/MWT_1.3.0_r1035/MultiWorm Tracker v1.3.0/data/MWT.dll" fn="MWT_reportImageCorrectionAlgorithm"("handle"=w437) -> ("return type"=w439:i32)  [unwired: 4 in, 2 out]
      n407 = Bundle("Value"=w493, "Value"=w492, "Value"=w491) -> (w490:T42)  [unwired: 1 in]
      n408 = local read "Image"() -> (w498:T3)
      n409 = property on="Tap" class="Bool (strict)"() -> ("Value"=w472:bool)  [unwired: 2 in, 2 out]
      n410 = Round To Nearest(number=w505) -> (nearest integer value=w507:dbl)
      n411 = Round To Nearest(number=w506) -> (nearest integer value=w508:dbl)
      n412 = Array Size(array=w433) -> (size(s)=w434:i32)
      n413 = Array Size(array=w429) -> (size(s)=w430:i32)
      n414 = Array Size(array=w431) -> (size(s)=w432:i32)
      n415 = Greater Than 0?(x=w439) -> (x > 0?=w438:bool)
      n416 = Array Size(array=w435) -> (size(s)=w436:i32)
      n417 = Bundle("Value"=w489, "Value"=w488) -> (w487:cluster{"Value":sgl[][], "Value":i32[][]})  [unwired: 1 in]
      n418 = Bundle("Value"=w456, "Value"=w455) -> (w457:cluster{"Value":sgl[][], "Value":i32[][]})  [unwired: 1 in]
      n419 = Bundle("Value"=w476, "Value"=w477) -> (w475:cluster{"Value":sgl[][], "Value":i32[][]})  [unwired: 1 in]
      n420 = call "IMAQ Create"("Image Name"="display") -> ("New Image"=w513:T3)  [unwired: 4 in, 1 out]
      n421 = To Long Integer(number=w507) -> (32bit integer=w503:i32)
      n422 = To Long Integer(number=w508) -> (32bit integer=w502:i32)
      n423 = case shown="True" w438 {
        tunnel: [i32[] [] w516] -> w440
        frame False {
        }
        frame True {
          n424 = Initialize Array(-1 ("element"), 200 ("dimension size")) -> (w516:i32[])
        }
      }
      n425 = call "IMAQ Copy"("Image Dst"=w513, "Image Src"=w498) -> ("Image Dst Out"=w450:T3)  [unwired: 4 in, 1 out]
      n426 = property on="Puff" class="Bool (strict)"() -> ("Value"=w471:bool)  [unwired: 2 in, 2 out]
      n427 = Initialize Array(i16 0 ("element"), w503, w502) -> (w499:i16[][])
      n428 = property on="Custom 2" class="Bool (strict)"() -> ("Value"=w459:bool)  [unwired: 2 in, 2 out]
      n429 = property on="Custom 1" class="Bool (strict)"() -> ("Value"=w470:bool)  [unwired: 2 in, 2 out]
      n430 = call "Init_Data_array.vi"() -> ("Data Cluster"=w509:T43)
      n431 = call "IMAQ GetImageSize"("Image"=w450) -> ("Y Resolution"=w453:i32, "X Resolution"=w452:i32)  [unwired: 3 in, 1 out]
      n432 = while {
        tunnel: w498 -> [w670]
        shift-right: [w636] -> _
        shift-left: w464 -> [w674]
        tunnel: w435 -> [w723]
        shift-right: [w718] -> _
        shift-left: 0 -> [w722]
        tunnel: w472 -> [w720]
        tunnel: w436 -> [w721]
        tunnel: w464 -> [w675]
        shift-right: [w725] -> _
        shift-left: 0 -> [w719]
        shift-right: [w696] -> _
        shift-left: 0 -> [w676]
        shift-right: [w695] -> _
        shift-left: w509 -> [w701]
        tunnel: w434 -> [w714]
        shift-right: [w708] -> _
        shift-left: 0 -> [w710]
        tunnel: w471 -> [w713]
        shift-right: [w707] -> _
        shift-left: 0 -> [w712]
        tunnel: w433 -> [w715]
        tunnel: w490 -> [w633]
        tunnel: w487 -> [w624]
        tunnel: w478 -> [w699]
        tunnel: w475 -> [w622]
        shift-right: [w685] -> _
        shift-left: 0 -> [w693]
        shift-right: [w684] -> _
        shift-left: 0 -> [w690]
        tunnel: w432 -> [w692]
        tunnel: w470 -> [w691]
        tunnel: w431 -> [w694]
        shift-right: [w683] -> _
        shift-left: 1 -> [w669]
        shift-right: [w678] -> _
        shift-left: 0 -> [w682]
        shift-right: [w677] -> _
        shift-left: w499 -> [w677]
        shift-right: [w666] -> w466
        shift-left: w462 -> [w664]
        tunnel: w457 -> [w616]
        shift-right: [w656] -> _
        shift-left: 0 -> [w660]
        shift-right: [w657] -> _
        shift-left: 0 -> [w663]
        tunnel: w430 -> [w661]
        tunnel: w459 -> [w662]
        tunnel: w429 -> [w651]
        tunnel: w453 -> [w641]
        tunnel: w452 -> [w640]
        tunnel: w450 -> [w639]
        shift-right: [w631] -> _
        shift-left: 0 -> [w635]
        shift-right: [w630] -> _
        shift-left: 0 -> [w634]
        shift-right: [w627] -> _
        shift-left: 0 -> [w629]
        shift-right: [w626] -> _
        shift-left: 0 -> [w628]
        shift-right: [w619] -> _
        shift-left: 0 -> [w621]
        shift-right: [w618] -> _
        shift-left: 0 -> [w620]
        shift-right: [w613] -> _
        shift-left: 0 -> [w615]
        shift-right: [w612] -> _
        shift-left: 0 -> [w614]
        shift-right: [w610] -> _
        shift-left: 0 -> [w611]
        shift-right: [w608] -> _
        shift-left: w440 -> [w609]
        stop <- w603 stop-if-true
        # "Elapsed time\nCurrent time\ntime since last frame"
        # "Event is a bitmask"
        # "Custom 1 Stimuli"
        # "Mark Stimulus event"
        # "Retrieve statisical data in to the graphs"
        # "Custom 2 Stimuli"
        # "Puff Stimuli"
        # "Tap stimuli"
        # "Run the actual experiment."
        n433 = call "get_time.vi"("input cluster"=w664) -> ("millisecond timer value"=w636:u32)
        n434 = Subtract(x=w636, y=w675) -> (x-y=w607:u32)
        n435 = Divide(x=w607, y=sgl 1000.0) -> (x/y=w648:sgl)
        n436 = property on="User interface display slector" class="Ring (strict)"() -> ("Value"=w602:u16)  [unwired: 2 in, 2 out]
        n437 = call "GetStimulusArrayValues.vi"("tap train index"=w611, "time between onset index"=w634, "fraction of time between index"=w635, "Cluster"=w633, "time since beginning of run"=w607) -> ("tap train index out"=w610:i32, "time between onset index out"=w630:i32, "fraction of time between index out"=w631:i32, "stimulus settings"=w632:cluster{"outy3":sgl, "outy3":i32, "Value":i32})
        n438 = call "GetOtherStimulusArrayValues.vi"("time between onset index"=w620, "fraction of time between index"=w621, "Cluster"=w622, "time since beginning of run"=w607) -> ("time between onset index out"=w618:i32, "fraction of time between index out"=w619:i32, "stimulus settings"=w623:cluster{"outy3":sgl, "outy3":i32})
        n439 = call "GetOtherStimulusArrayValues.vi"("time between onset index"=w614, "fraction of time between index"=w615, "Cluster"=w616, "time since beginning of run"=w607) -> ("time between onset index out"=w612:i32, "fraction of time between index out"=w613:i32, "stimulus settings"=w617:cluster{"outy3":sgl, "outy3":i32})
        n440 = call "GetOtherStimulusArrayValues.vi"("time between onset index"=w628, "fraction of time between index"=w629, "Cluster"=w624, "time since beginning of run"=w607) -> ("time between onset index out"=w626:i32, "fraction of time between index out"=w627:i32, "stimulus settings"=w625:cluster{"outy3":sgl, "outy3":i32})
        n441 = case shown="0, Default" w602 {
          frame 0, Default {
            w733 = u16 0 items=["Raw Image", "Memory Image", "Fixed Image"] ("What to display")
            n442 = property on="Display/Don't Display" class="Bool (strict)"("Value"=TRUE ("Display/Don't Display")) -> ()  [unwired: 2 in, 2 out]
            n443 = property on="What to display" class="Ring (strict)"("Value"=w733) -> ()  [unwired: 2 in, 2 out]
          }
          frame 1 {
            w735 = u16 1 items=["Raw Image", "Memory Image", "Fixed Image"] ("What to display")
            n444 = property on="Display/Don't Display" class="Bool (strict)"("Value"=TRUE ("Display/Don't Display")) -> ()  [unwired: 2 in, 2 out]
            n445 = property on="What to display" class="Ring (strict)"("Value"=w735) -> ()  [unwired: 2 in, 2 out]
          }
          frame 2 {
            w737 = u16 2 items=["Raw Image", "Memory Image", "Fixed Image"] ("What to display")
            n446 = property on="Display/Don't Display" class="Bool (strict)"("Value"=TRUE ("Display/Don't Display")) -> ()  [unwired: 2 in, 2 out]
            n447 = property on="What to display" class="Ring (strict)"("Value"=w737) -> ()  [unwired: 2 in, 2 out]
          }
          frame 3 {
            w739 = u16 2 items=["Raw Image", "Memory Image", "Fixed Image"] ("What to display")
            n448 = property on="Display/Don't Display" class="Bool (strict)"("Value"=FALSE ("Display/Don't Display")) -> ()  [unwired: 2 in, 2 out]
            n449 = property on="What to display" class="Ring (strict)"("Value"=w739) -> ()  [unwired: 2 in, 2 out]
          }
        }
        n450 = call "elapsed_time.vi"("Time since last update"=w682, "Initial Time"=w674, "Current Time"=w636) -> ("Elapsed Time"=w679:i32)
        n451 = Bundle("custom timing array"=w694, w693, w692, "Value"=w691, w690, "stimulus settings"=w623) -> (w689:T44)  [unwired: 1 in]
        n452 = Bundle("custom 2 timing array"=w651, w660, w661, "Value"=w662, w663, "stimulus settings"=w617) -> (w653:T45)  [unwired: 1 in]
        n453 = property on="Minimum time between events(ms)" class="DigNum (strict)"() -> ("Value"=w606:u32)  [unwired: 2 in, 2 out]
        n454 = Unbundle(w664) -> (w668:T19)  [unwired: 1 out]
        n455 = property on="last acquired buffer" class="DigNum (strict)"() -> ("Value"=w667:i32)  [unwired: 2 in, 2 out]
        n456 = Bundle("puff timing array"=w715, w710, w714, "Value"=w713, w712, "stimulus settings"=w625) -> (w716:T46)  [unwired: 1 in]
        n457 = control-ref of="Time until Next Puff"() -> (w717:refnum<vi>)
        n458 = control-ref of="Time until Next Custom 2"() -> (w654:refnum<vi>)
        n459 = control-ref of="Time until Next Custom 1"() -> (w688:refnum<vi>)
        n460 = Bundle(w668, "Value"=w667) -> (w666:T36)  [unwired: 1 in]
        n461 = property on="Display/Don't Display" class="Bool (strict)"() -> ("Value"=w642:bool)  [unwired: 2 in, 2 out]
        n462 = control-ref of="Time until Next Tap"() -> (w728:refnum<vi>)
        n463 = property on="Seconds into Experiment" class="DigNum (strict)"("Value"=w648) -> ()  [unwired: 2 in, 2 out]
        n464 = Bundle("tap timing array"=w723, w722, w721, "Value"=w720, w719, "stimulus settings"=w632) -> (w724:T47)  [unwired: 1 in]
        n465 = Bundle(w607, "millisecond timer value"=w636, "millisecond timer value"=w674, "Value"=w606) -> (w655:T48)  [unwired: 1 in]
        n466 = call "smart_get.vi"("Input Image"=w670, "Cluster"=w666) -> ("Image Out"=w644:T3, "Acquired Buffer Number"=w665:i32)
        n467 = property on="Tracker Handle" class="DigNum (strict)"() -> ("Value"=w700:i32)  [unwired: 2 in, 2 out]
        n468 = case shown="True" w642 {
          tunnel: [i16[][] [] ("Image Pixels (I16)") w748] -> w643
          tunnel: w641 -> [_ w745]
          tunnel: w640 -> [_ w744]
          frame False {
          }
          frame True {
            n469 = property on="Image Binning" class="Ring (strict)"() -> ("Value"=w743:u16)  [unwired: 2 in, 2 out]
            n470 = Divide(x=w745, y=w743) -> (x/y=w750:dbl)
            n471 = Divide(x=w744, y=w743) -> (x/y=w751:dbl)
            n472 = Round To Nearest(number=w750) -> (nearest integer value=w752:dbl)
            n473 = Round To Nearest(number=w751) -> (nearest integer value=w753:dbl)
            n474 = To Long Integer(number=w752) -> (32bit integer=w747:i32)
            n475 = To Long Integer(number=w753) -> (32bit integer=w746:i32)
            n476 = Initialize Array(i16 0 ("element"), w747, w746) -> (w748:i16[][])
          }
        }
        n477 = Greater?(x=w679, y=1000) -> (0:w681:bool)
        n478 = Bundle(w655, "Time until Next Tap"=w728, w724) -> (w727:T49)  [unwired: 1 in]
        n479 = Bundle(w655, "Time until Next Puff"=w717, w716) -> (w709:T50)  [unwired: 1 in]
        n480 = Bundle(w655, "Time until Next Custom 1"=w688, w689) -> (w687:T51)  [unwired: 1 in]
        n481 = Bundle(w655, "Time until Next Custom 2"=w654, w653) -> (w652:T52)  [unwired: 1 in]
        n482 = Bundle("millisecond timer value"=w636, "millisecond timer value"=w674, w676, w648, "Data Cluster"=w701, "Value"=w700, w699) -> (w698:T53)  [unwired: 1 in]
        n483 = case shown="True" w681 {
          tunnel: w669 -> [w755 w759]
          tunnel: [w754 1] -> w683
          tunnel: w679 -> [w756 w762]
          tunnel: [w756 0] -> w678
          frame False {
            n484 = Increment(x=w755) -> (x+1=w754:i32)
          }
          frame True {
            n485 = Divide(x=1000 ("y"), y=w762) -> (x/y=w760:dbl)
            n486 = Divide(x=w760, y=w759) -> (x/y=→"seconds per frame":dbl)
          }
        }
        n487 = property on="last acquired buffer" class="DigNum (strict)"("Value"=w665) -> ()  [unwired: 2 in, 2 out]
        n488 = call "puff_stimulus_generator.vi"("input cluster"=w709) -> ("output cluster"=w711:cluster{i32, i32, "Elapsed Time":i32})
        n489 = call "custom_1_stimulus_generator.vi"("input cluster"=w687) -> ("output cluster"=w686:cluster{i32, i32, "Elapsed Time":i32})
        n490 = call "custom_2_stimulus_generator.vi"("input cluster"=w652) -> ("output cluster"=w659:cluster{i32, i32, "Elapsed Time":i32})
        n491 = call "tap_stimulus_generator.vi"("input cluster"=w727) -> ("output cluster"=w726:T54)
        n492 = Unbundle(w711) -> (w672:i32, w708:i32, "Elapsed Time"=w707:i32)
        "# Puffs Delivered" <- w708
        n493 = Unbundle(w686) -> (w671:i32, w685:i32, "Elapsed Time"=w684:i32)
        "# Custom 1's Delivered" <- w685
        n494 = Unbundle(w659) -> (w658:i32, w656:i32, "Elapsed Time"=w657:i32)
        "# Custom 2's Delivered" <- w656
        n495 = call "graph_data_acquisition_and_display.vi"("input cluster"=w698) -> ("output cluster"=w697:T55)
        n496 = Unbundle(w726) -> (w673:i32, "Tap Number"=w718:i32, "Elapsed Time"=w725:i32)
        "# Taps Delivered" <- w718
        n497 = property on="Tracker Handle" class="DigNum (strict)"() -> ("Value"=w650:i32)  [unwired: 2 in, 2 out]
        n498 = property on="Image Binning" class="Ring (strict)"() -> ("Value"=w649:u16)  [unwired: 2 in, 2 out]
        n499 = property on="What to display" class="Ring (strict)"() -> ("Value"=w647:u16)  [unwired: 2 in, 2 out]
        n500 = property on="Display/Don't Display" class="Bool (strict)"() -> ("Value"=w645:bool)  [unwired: 2 in, 2 out]
        n501 = property on="Image Bit Depth" class="DigNum (strict)"() -> ("Value"=w646:u32)  [unwired: 2 in, 2 out]
        n502 = property on="Seconds into Experiment" class="DigNum (strict)"() -> ("Value"=w702:dbl)  [unwired: 2 in, 2 out]
        n503 = property on="Experiment Duration (s)" class="DigNum (strict)"() -> ("Value"=w730:dbl)  [unwired: 2 in, 2 out]
        n504 = Unbundle(w697) -> ("Elapsed Time"=w696:i32, "Data Cluster"=w695:T43)
        n505 = formula code="int32 event = 0b0;\nif( e1 > 0 ) \n  event += 0b0001;\nif( e2 > 0 ) \n  event += 0b0010;\nif( e3 > 0 )\n  event += 0b0100;\nif( e4 > 0 )\n  event += 0b1000;"("e1"=w673, "e2"=w672, "e3"=w671, "e4"=w658) -> ("event"=w638:i32)
        n506 = Greater Or Equal?(x=w702, y=w730) -> (x >= y?=w604:bool)
        n507 = Greater Than 0?(x=w730) -> (x > 0?=w605:bool)
        n508 = And(x=w604, y=w605) -> (x .and. y?=w729:bool)
        n509 = property on="Stop" class="Bool (strict)"() -> ("Value"=w731:bool)  [unwired: 2 in, 2 out]
        n510 = Bundle(w638, "Value"=w650, "Value"=w649, w648, "Value"=w647, "Value"=w645, "Value"=w646, "Image Out"=w644, "Image Pixels (I16)"=w643, w609) -> (w637:T56)  [unwired: 1 in]
        n511 = Or(x=w729, y=w731) -> (x .or. y?=w603:bool)
        n512 = property on="Proccessing loop stopped?" class="Bool (strict)"("Value"=w603) -> ()  [unwired: 2 in, 2 out]
        n513 = call "processing_steps.vi"("input cluster"=w637) -> ("output cluster"=w706:T57)
        n514 = Unbundle(w706) -> ("return value"=w705:i32, "return value"=→"error count":i32, "Image Pixels (I16) out"=w703:i16[][], "coordinates"=w608:i32[])
        n515 = case shown="True" w603 {
          frame False {
          }
          frame True {
            n516 = property on="Stop" class="Bool (strict)"("Value"=TRUE ("Stop")) -> ()  [unwired: 2 in, 2 out]
          }
        }
        n517 = case shown="True" w645 {
          tunnel: w703 -> [_ w771]
          tunnel: w639 -> [_ w766]
          frame False {
          }
          frame True {
            n518 = property on="Image Bit Depth" class="DigNum (strict)"() -> ("Value"=w768:u32)  [unwired: 2 in, 2 out]
            n519 = call "IMAQ ArrayToImage"("Image Pixels (I16)"=w771, "Image"=w766) -> ("error out"=w764:errorcluster, "Image Out"=w770:T3)  [unwired: 8 in]
            n520 = call "IMAQ Image Bit Depth"("Image"=w770, "Bit Depth (0)"=w768, "error in (no error)"=w764, "Get/Set Bit Depth? (Set)"=TRUE) -> ("Image Out"=w769:T3, "error out"=→"error out 2":errorcluster)  [unwired: 9 in, 1 out]
            n521 = local write "Image"(w769) -> ()
          }
        }
        n522 = property on="Objects Found" class="DigNum (strict)"("Value"=w705) -> ()  [unwired: 2 in, 2 out]
      }
    }
    frame #6 {
      w775 = TRUE ("Make Available")
      # "Finalization, including cleanup and \nrestoration of initial control state."
      # "MWT_complete"
      # "MWT_killHandle"
      n523 = property on="Tracker Handle" class="DigNum (strict)"() -> ("Value"=w778:i32)  [unwired: 2 in, 2 out]
      n524 = call "camera_closer.vi"("input cluster"=w774) -> ()
      n525 = Unbundle(w776) -> (w773:T10, w772:T9)  [unwired: 1 out]
      n526 = dll-call lib="C:/Users/Marc/multi worm tracker/MWT_1.3.0_r1035/MultiWorm Tracker v1.3.0/data/MWT.dll" fn="MWT_complete"("handle"=w778) -> ("handle"=w779:i32)  [unwired: 4 in, 2 out]
      n527 = Cluster To Array(cluster=w772) -> (array=w777:refnum<vi>[])
      n528 = call "make_buttons_available.vi"("array"=w777, "Make Available"=w775) -> ()
      n529 = dll-call lib="C:/Users/Marc/multi worm tracker/MWT_1.3.0_r1035/MultiWorm Tracker v1.3.0/data/MWT.dll" fn="MWT_killHandle"("handle"=w779) -> ()  [unwired: 5 in, 2 out]
      n530 = call "make_controls_available.vi"("input cluster"=w773, "Make Available"=w775) -> ()
    }
  }
  "Objects Found" <- w24
  "Seconds into Experiment" <- w24
  "Time until Next Puff" <- w24
  "Time until Next Tap" <- w24
  "First-call" <- TRUE ("First-call")
  "Proccessing loop stopped?" <- FALSE ("Proccessing loop stopped?")
  "Image" <- T3 refnum ("Image")
  "XY Graph" <- w3
  "XY Graph 2" <- w3
  "XY Graph 3" <- w3
  "XY Graph 4" <- w3
  "Time until Next Custom 1" <- w24
  "Auto-start in (s)" <- w24
  "Time until Next Custom 2" <- w24
